vi "SDK Sample_modified.vi"() -> ()   [LabVIEW 2015]
uses:
  sub/Mode.ctl
  sub/global.vi
panel:
  out "Error?":bool
  out "size(s)":i32
  out "Data(8Bit)":u8[](array[numeric])
  out "Data(16Bit)":u16[](array[numeric])
  out "Depth":i8
  out "nDeviceNoList":u32[](array[numeric])
  out "MaxSize":cluster{"pWidth":u32, "pHeight":u32}={"pWidth"=2048, "pHeight"=2048}
  out "pDetectNumInfoLV":T1
  out "SetupCover2":string
  out "SetupCover1":string
  out "FLG_LiveStop":u16(ring) items=["Live", "Get", "Stop"]
  in  "Variable":bool caption="Calibrate"
  in  "Record Option":bool caption="Calibrate"
  in  "Update:":u16(ring) items=["OFF", "ON"]
  in  "Low  Light:":u16(ring) items=["OFF", "ON"]
  in  "Save Setup":bool caption="Calibrate"
  out "RetryCount":u8
  out "FLG_LiveStop":bool
  out "ColorType":enum16{"MONO", "COLOR"}(ring)
  out "Frame":i32(slide) scale=-2046.0..2045.0
  out "RecordStatus":u16(ring) items=["Record", "WaitingTRG", "Endless", "Recording"]
  out "Resolution":cluster{"pWidth":u32, "pHeight":u32}
  out "Picture":picture
  out "Mode":T2=enum."Error"
  out "Out_IP Address":T3 caption="Info_IP Address" {"Manual_IP"."IP4" format="%.03d"; "Manual_IP"."IP3" format="%.03d"; "Manual_IP"."IP2" format="%.03d"; "Manual_IP"."IP1" format="%.03d"; "Auto_IP"."IP3" format="%.03d"; "Auto_IP"."IP2" format="%.03d"; "Auto_IP"."IP1" format="%.03d"}
  out "nInterfaceCode":u32 format="%.0x"
  in  "stop":bool caption="停止"
  in  "Tab":enum32{"Camera", "Data Save", "File View"}(tab)
  in  "Record":bool caption="Calibrate"
  in  "RecStop":bool caption="Calibrate"
  in  "Setup":T4={"Frame Rate:"=0, "Shutter:"=0, "Resolution:"=4, "Trigger Mode:"=0, "Shading:"=0, "Partition:"=1, "Camera Option"=FALSE, "CameraInfo"={"Head:"=0, "Camera:"=0}} {"CameraInfo"."Camera:" items=["FASTCAM SA4 model 500K-M1"]; "CameraInfo"."Head:" items=["Head No.1"]; "Shading:" items=["Shading"]; "Shutter:" items=["1/50 sec", "1/60 sec", "1/100 sec", "1/200 sec", "1/300 sec", "1/400 sec", "1/500 sec", "1/600 sec", "1/700 sec", "1/800 sec", "1/900 sec", "1/1000 sec", "1/2000 sec", "1/3000 sec", "1/4000 sec", "1/5000 sec", "1/6000 sec", "1/7000 sec", "1/8000 sec", "1/9000 sec", "1/10000 sec", "1/12000 sec", "1/15000 sec", "1/17000 sec", "1/20000 sec", "1/25000 sec", "1/30000 sec", "1/34000 sec", "1/39000 sec", "1/50000 sec", "1/57000 sec", "1/62000 sec", "1/74000 sec", "1/82000 sec", "1/92000 sec", "1/104000 sec", "1/178000 sec", "1/333000 sec", "1/593000 sec", "1/1000000 sec"]; "Trigger Mode:" items=["START", "CENTER", "END", "MANUAL", "RANDOM", "RANDOM_RESET", "RANDOM_CENTER", "RANDOM_MANUAL", "TWOSTAGE_1/2", "TWOSTAGE_1/4", "TWOSTAGE_1/8"]; "Frame Rate:" items=["50 fps", "60 fps", "125 fps", "250 fps", "500 fps", "1000 fps", "2000 fps", "3000 fps", "3600 fps", "4500 fps", "5000 fps", "6000 fps", "6750 fps", "8000 fps", "10000 fps", "13500 fps", "20000 fps", "30000 fps", "40000 fps", "50000 fps", "60000 fps", "75000 fps", "86400 fps", "100000 fps", "150000 fps", "225000 fps", "360000 fps", "500000 fps"]; "Resolution:" items=["1024 X 1024", "1024 X 896", "1024 X 800", "1024 X 640", "1024 X 512", "896 X 896", "896 X 752", "896 X 640", "896 X 512", "768 X 768", "768 X 640", "768 X 512", "640 X 640", "512 X 512", "512 X 384", "512 X 352", "384 X 288", "320 X 240", "320 X 192", "320 X 160", "320 X 128", "256 X 256", "256 X 128", "256 X 64", "192 X 128", "128 X 128", "128 X 96", "128 X 64", "128 X 32", "128 X 16", "64 X 16"]; "Partition:" items=["Partition 1"=1]}
  in  "Display:":enum32{"Live", "Mem", "LiveStop"}(radio)
  in  "DataSaveInfo":T5={"DS-Format"=2, "DS-File name:"="", "DS-Save Path"=path "", "DS-Head"=0, "DS-Save"=FALSE, "Data_Slide"=0, "PLAY"=FALSE, "STOP"=FALSE, "StartFrame"=0, "EndFrame"=0, "CurrentFrame"=0, "DS-Camera:"=0} {"DS-Camera:" items=["FASTCAM SA4 model 500K-M1"]; "CurrentFrame" min=-2046 max=8871 step=1; "EndFrame" min=-2046 max=8871 step=1; "StartFrame" min=-2046 max=8871 step=1; "Data_Slide" scale=-2046.0..8871.0; "DS-Head" items=["Head No.1"]; "DS-Format" items=["BMP", "JPEG", "AVI"]}
  # "．"
  # "．"
  # "．"
  # "．"
  # "．"
  # "．"
  # "XXX"
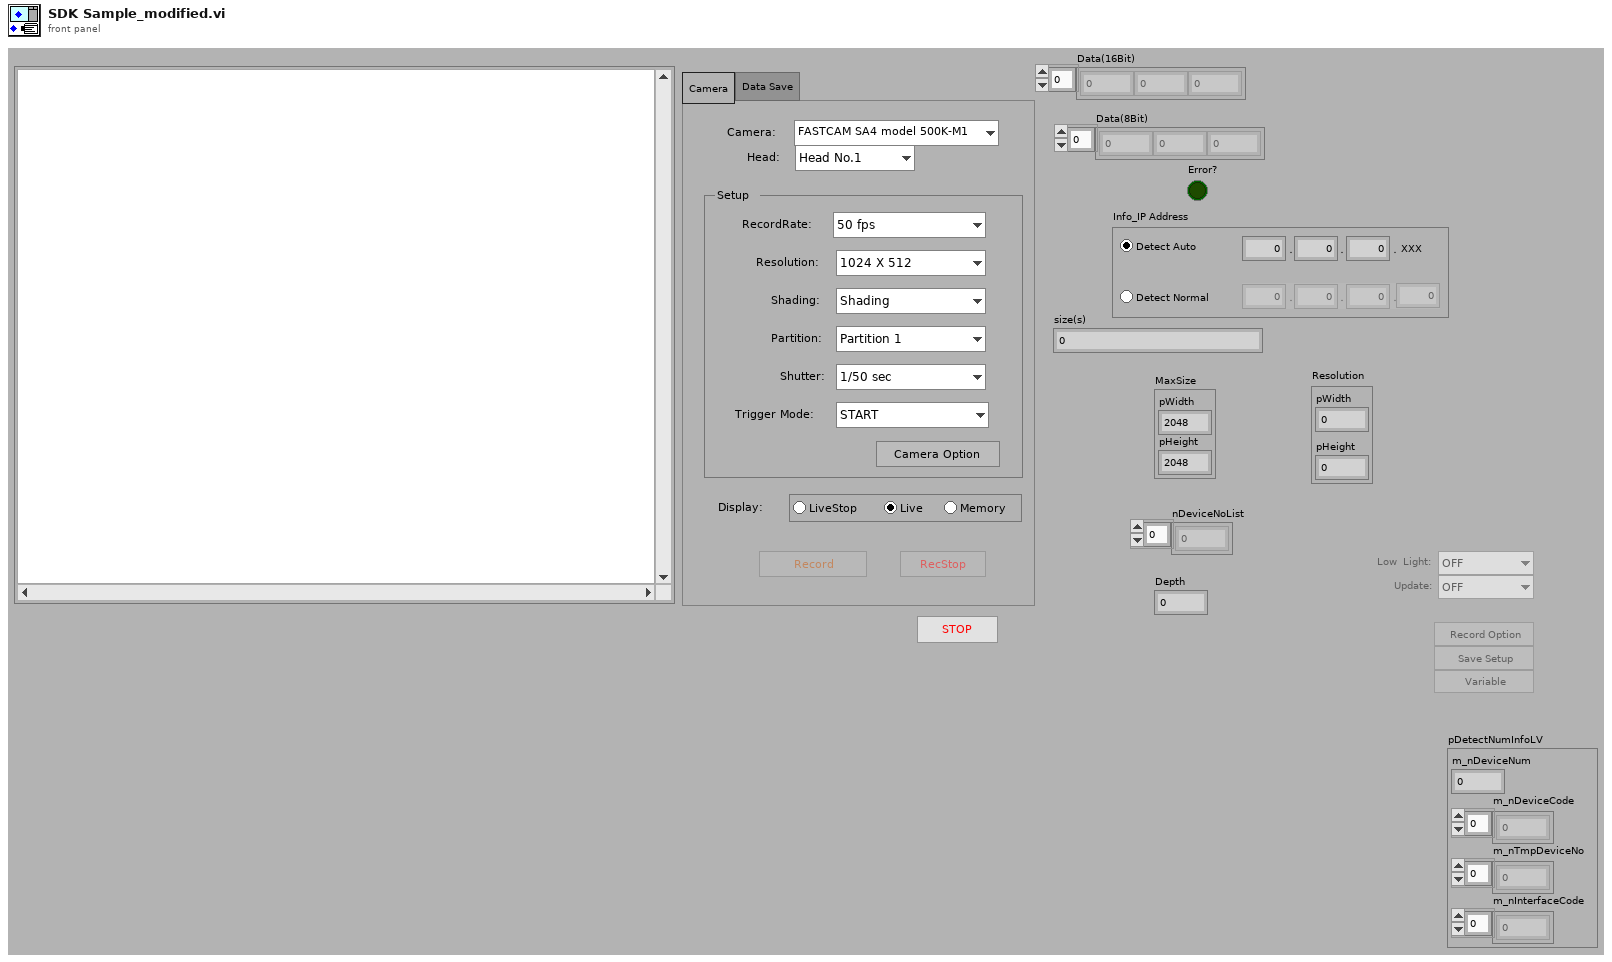
[diagram p1: front panel]
types:
  T1 = cluster{"m_nDeviceNum":u32, "m_nDeviceCode":u32[], "m_nTmpDeviceNo":u32[], "m_nInterfaceCode":u32[]}
  T2 = typedef "Mode.ctl" = enum16{"Default", "Error", "End", "Init", "DetectDevice", "Open", "Close", "GetDeviceName", "GetExistChildDeviceList", "GetColorType", "GetBitDepth.vi", "GetRecordRateList", "GetRecordRate", "SetRecordRate", "GetShutterSpeedFpsList", "GetShutterSpeedFps", "SetShutterSpeedFps", "GetResolutionList", "GetResolution", "SetResolution", "GetTriggerModeList", "GetTriggerMode", "SetTriggerMode", "GetPartitionList", "SetPartitionList", "GetCurrentPartition", "SetCurrentPartition", "GetShadingModeList", "DataSave"}
  T3 = cluster{"Detect Select BOX":enum32{"Detect Auto", "Detect Normal"}, "Auto_IP":cluster{"IP1":u8, "IP2":u8, "IP3":u8}, "Manual_IP":cluster{"IP1":u8, "IP2":u8, "IP3":u8, "IP4":u8}}
  T4 = cluster{"Frame Rate:":u16, "Shutter:":u16, "Resolution:":u16, "Trigger Mode:":u16, "Shading:":u16, "Partition:":u16, "Camera Option":bool, "CameraInfo":cluster{"Head:":u16, "Camera:":u16}}
  T5 = cluster{"DS-Format":u16, "DS-File name:":string, "DS-Save Path":path, "DS-Head":u16, "DS-Save":bool, "Data_Slide":i32, "PLAY":bool, "STOP":bool, "StartFrame":i32, "EndFrame":i32, "CurrentFrame":i32, "DS-Camera:":u16}
  T6 = enum32{"Page Enabled", "Page Disabled", "Page Disabled & Grayed"}
  T7 = cluster{"return type":u32, "pErrorCode":u32, "error ":errorcluster}
  T8 = cluster{"ReturnValue":u32, "ErrorCode":u32, "error ":errorcluster}
  T9 = cluster{"Start":i32, "End":i32, "Trigger":i32, "TwoStageLowToHigh":i32, "TwoStageHighToLow":i32, "TwoStageTiming":u32, "Event":i32[], "EventCount":u32, "RecordedFrames":u32}
  T10 = typedef "imagedata.ctl" = cluster{"image type":i32, "image depth":i32, "image":u8[], "mask":u8[], "colors":u32[], "Rectangle":cluster{"left":i16, "top":i16, "right":i16, "bottom":i16}}
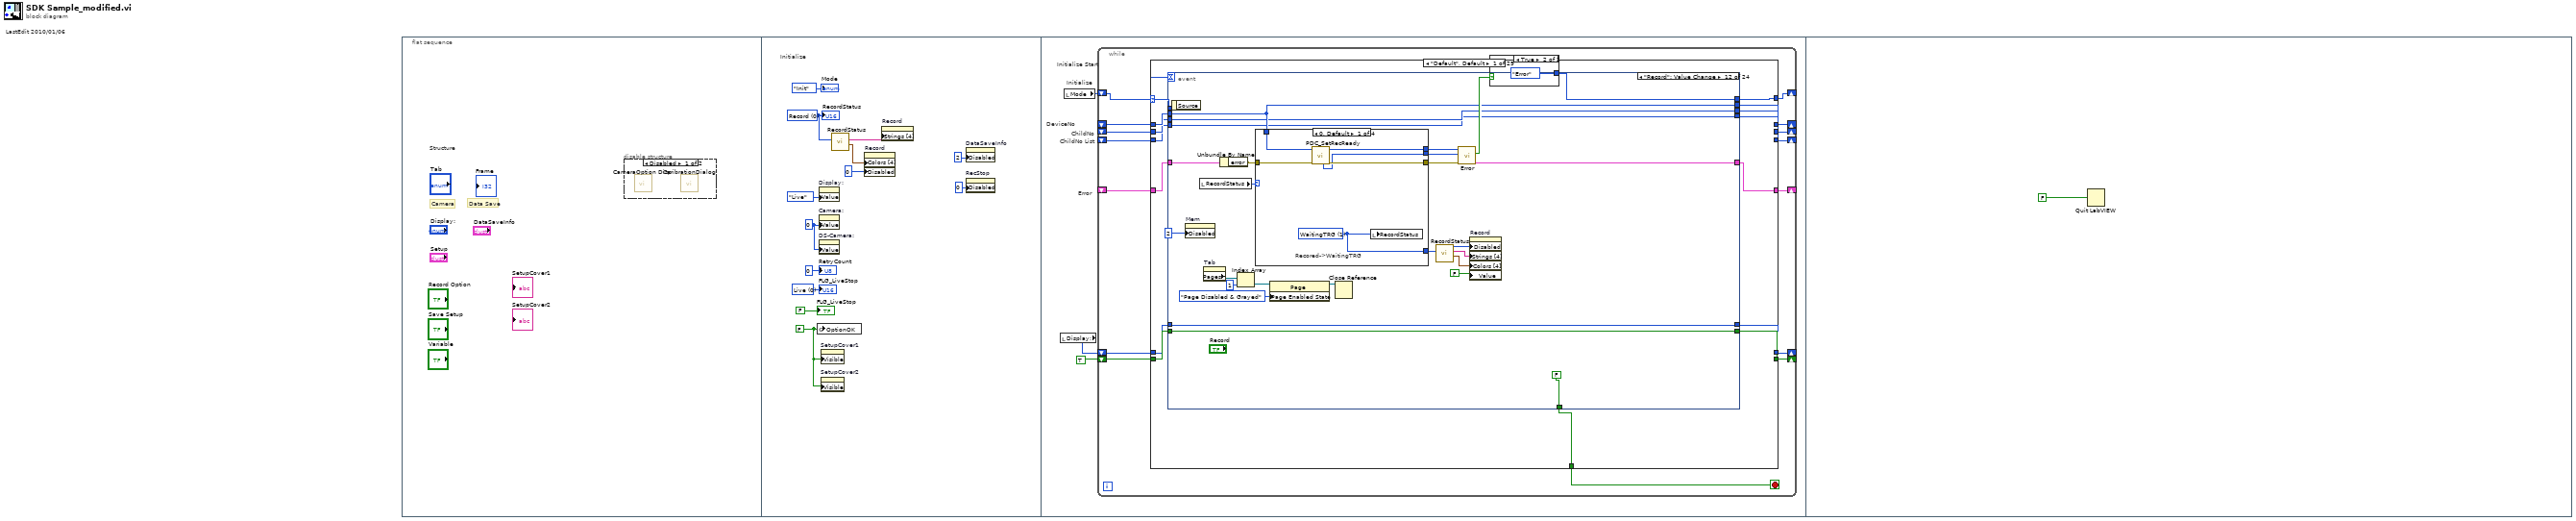
[diagram p0: block diagram]
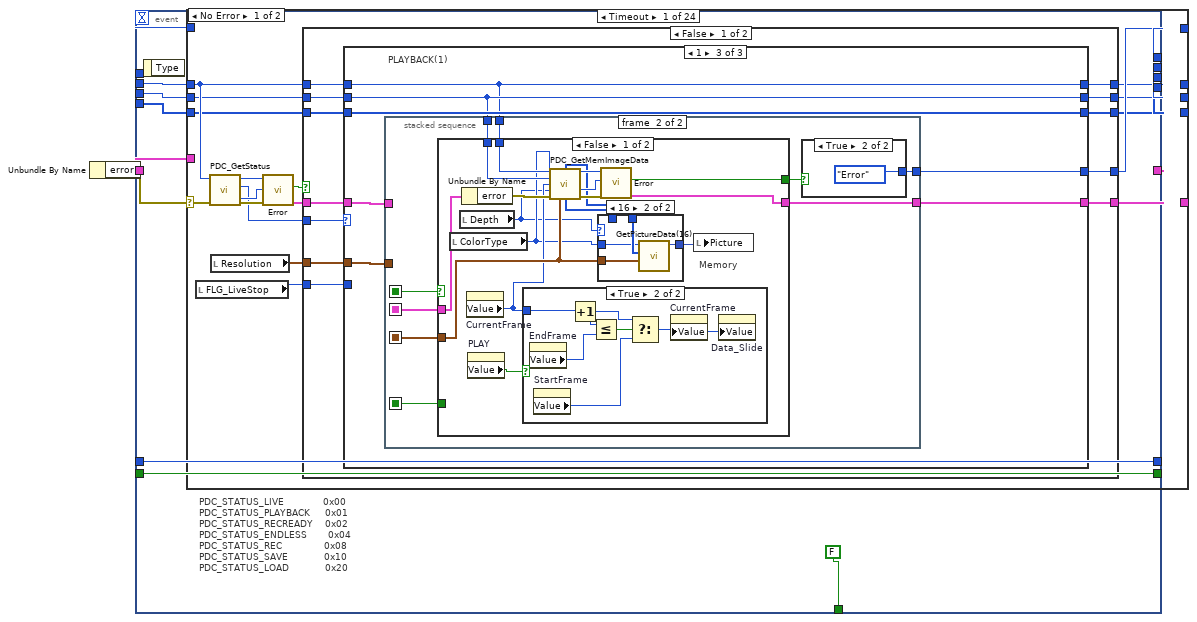
[diagram p3: hidden frame]
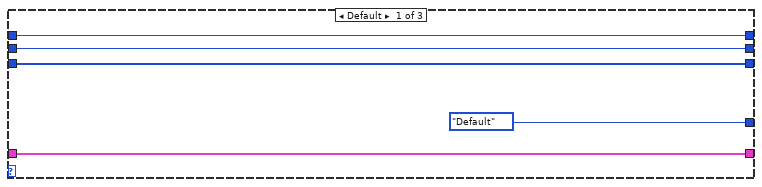
[diagram p4: hidden frame]
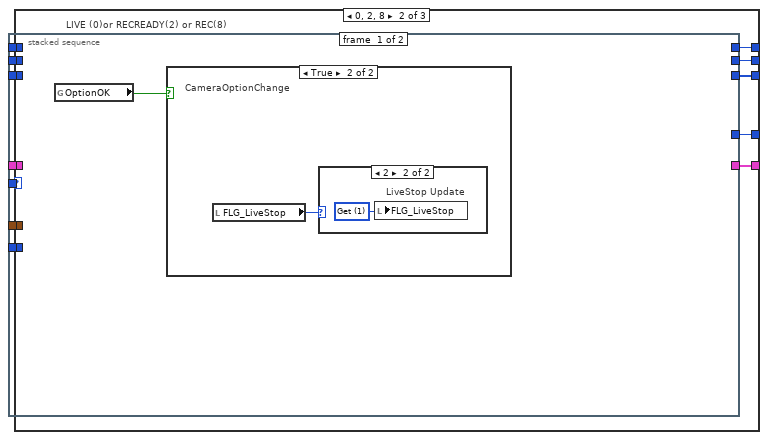
[diagram p5: hidden frame]
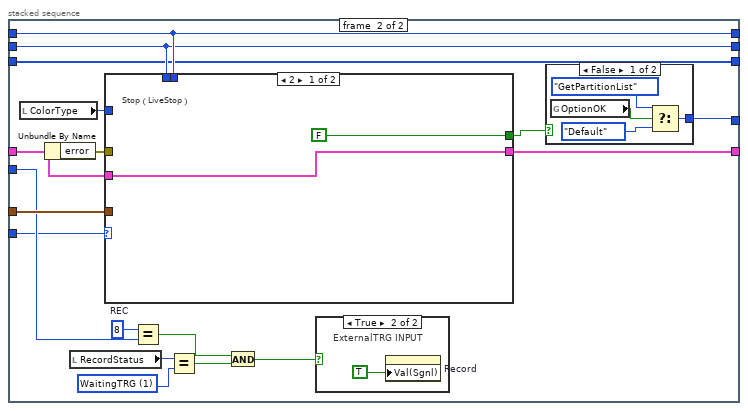
[diagram p8: hidden frame]
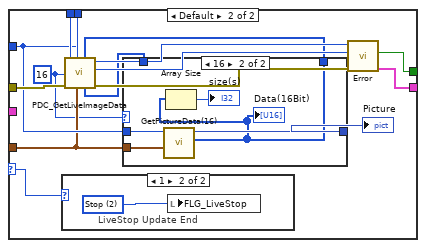
[diagram p10: hidden frame]
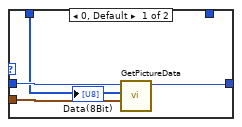
[diagram p11: hidden frame]
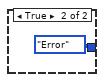
[diagram p13: hidden frame]
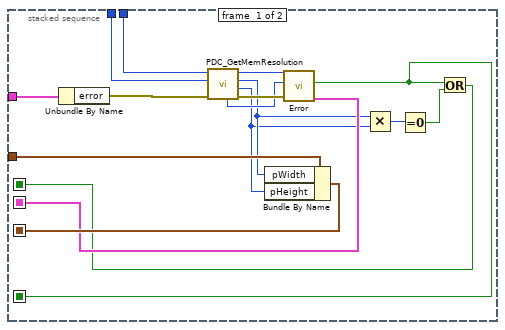
[diagram p14: hidden frame]
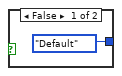
[diagram p15: hidden frame]
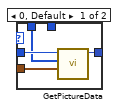
[diagram p16: hidden frame]
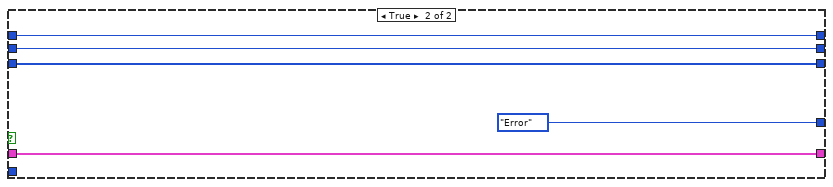
[diagram p19: hidden frame]
diagram:
  # "LastEdit 2010/01/06"
  n1 = flat-sequence {
    frame #0 {
      # "Structure"
      # "Camera"
      # "Data Save"
      n2 = disable-structure shown="Disabled" {
        frame Disabled {
          n3 = call "CameraOption Disp.vi"() -> ()  [unwired: 12 in]
          n4 = call "CaribrationDialog.vi"() -> ()  [unwired: 1 in]
        }
        frame Enabled {
        }
      }
    }
    frame #1 {
      w2 = u16 0 ("値")
      w3 = FALSE ("OptionOK")
      w4 = u16 0 items=["Live", "Get", "Stop"] ("FLG_LiveStop")
      w13 = u16 0 items=["Record", "WaitingTRG", "Endless", "Recording"] ("RecordStatus")
      # "Initialize"
      n5 = global write "global.vi" "OptionOK"(w3) -> ()
      n6 = property on="Display:" class="RadioBtnsControl (strict)"("Value"=enum32{"Live", "Mem", "LiveStop"}."Live" ("Display:")) -> ()  [unwired: 2 in, 2 out]
      n7 = property on="Camera:" class="Ring (strict)"("Value"=w2) -> ()  [unwired: 2 in, 2 out]
      n8 = property on="DS-Camera:" class="Ring (strict)"("Value"=w2) -> ()  [unwired: 2 in, 2 out]
      n9 = property on="SetupCover1" class="Str"("Visible"=w3) -> ()  [unwired: 2 in, 2 out]
      n10 = property on="SetupCover2" class="Str"("Visible"=w3) -> ()  [unwired: 2 in, 2 out]
      n11 = call "RecordStatus.vi"("RecordStatus"=w13) -> ("Color[4]"=w11:cluster{u32, u32}[], "String[4]"=w12:string[])  [unwired: 9 out]
      n12 = property on="Record" class="Bool (strict)"("Colors [4]"=w11, "Disabled"=u8 0 ("無効")) -> ()  [unwired: 2 in, 2 out]
      n13 = property on="Record" class="Bool (strict)"("Strings [4]"=w12) -> ()  [unwired: 2 in, 2 out]
      n14 = property on="DataSaveInfo" class="Clust (strict)"("Disabled"=u8 2 ("無効")) -> ()  [unwired: 2 in, 2 out]
      n15 = property on="RecStop" class="Bool (strict)"("Disabled"=u8 0 ("無効")) -> ()  [unwired: 2 in, 2 out]
      "Mode" <- Mode."Init" ("Mode")
      "RecordStatus" <- w13
      "FLG_LiveStop" <- FALSE ("FLG_LiveStop")
      "RetryCount" <- u8 0 ("RetryCount")
      "FLG_LiveStop" <- w4
    }
    frame #2 {
      # "Error"
      # "ChildNo List"
      # "Initialize"
      # "Initialize Start"
      # "ChildNo"
      # "DeviceNo"
      n16 = local read "Display:"() -> (w14:enum32{"Live", "Mem", "LiveStop"})
      n17 = local read "Mode"() -> (w16:T2)
      n18 = while {
        shift-right: [w29] -> _
        shift-left: w16 -> [w31]
        shift-right: [w27] -> _
        shift-left: _ -> [w28]
        shift-right: [w26] -> _
        shift-left: _ -> [w25]
        shift-right: [w24] -> _
        shift-left: _ -> [w23]
        shift-right: [w21] -> _
        shift-left: TRUE -> [w22]
        shift-right: [w20] -> _
        shift-left: _ -> [w19]
        shift-right: [w17] -> _
        shift-left: w14 -> [w18]
        stop <- w30 stop-if-true
        n19 = case shown="\"Default\", Default" w31 {
          selector: w31 -> [w40 _ _ _ _ _ _ _ _ _ _ _ _ _ _ _ _ _ _ _ _ _ _ _ _ _ _ _ _]
          tunnel: [w43 FALSE ("T button?") w733 FALSE ("T button?") FALSE ("T button?") FALSE ("T button?") TRUE ("T button?") FALSE ("T button?") FALSE ("T button?") FALSE ("T button?") FALSE ("T button?") FALSE ("T button?") FALSE ("T button?") FALSE ("T button?") FALSE ("T button?") FALSE ("T button?") FALSE ("T button?") FALSE ("T button?") FALSE ("T button?") FALSE ("T button?") FALSE ("T button?") FALSE ("T button?") FALSE ("T button?") FALSE ("T button?") FALSE ("T button?") FALSE ("T button?") FALSE ("T button?") FALSE ("T button?") FALSE ("T button?")] -> w30
          tunnel: w28 -> [w47 w730 w744 _ w837 w859 w894 w923 w953 w974 w991 w1012 w1040 w1065 w1088 w1118 w1142 w1171 w1207 w1240 w1260 w1283 w1301 w1335 w1357 w1379 w1391 w1418 w1467]
          tunnel: [w46 T7 {"return type"=1, "pErrorCode"=1, "error "={"status"=FALSE, "code"=0, "source"=""}} ("Error_Out") T7 {"return type"=1, "pErrorCode"=1, "error "={"status"=FALSE, "code"=0, "source"=""}} ("Error_Out") w778 w835 w858 w891 w915 w952 w972 w989 w1010 w1038 w1063 w1086 w1116 w1143 w1169 w1205 w1239 w1258 w1281 w1300 w1330 w1352 w1374 w1390 w1417 w1456] -> w27
          tunnel: [w44 Mode."Default" ("Mode") w732 w780 w838 w861 Mode."Default" ("Mode") w924 w955 w978 w995 w1016 w1044 w1069 w1092 w1122 w1144 w1175 w1211 w1237 w1264 w1286 w1299 w1329 w1351 w1373 w1394 w1403 w1454] -> w29
          tunnel: [w41 w710 w741 w774 w829 w857 w893 w921 w950 w970 w987 w1008 w1036 w1061 w1084 w1114 w1145 w1167 w1203 w1238 w1256 w1279 w1298 w1332 w1354 w1376 w1393 w1416 w1452] -> w26
          tunnel: w25 -> [w42 w710 w741 w774 w829 _ w893 w921 w950 w970 w987 w1008 w1036 w1061 w1084 w1114 w1145 w1167 w1203 w1238 w1256 w1279 w1298 w1332 w1354 w1376 w1393 w1416 w1463]
          tunnel: [w38 w711 w742 w777 w826 w856 w892 w920 w939 w966 w984 w1000 w1026 w1053 w1076 w1105 w1131 w1162 w1191 w1223 w1253 w1276 w1297 w1331 w1353 w1375 w1392 w1415 w1453] -> w24
          tunnel: w23 -> [w39 w711 w742 w777 w826 w856 w892 w920 _ w966 w984 w1000 w1026 w1053 w1076 w1105 w1131 w1162 w1191 w1223 w1253 w1276 w1297 w1331 w1353 w1375 w1392 w1415 w1468]
          tunnel: w22 -> [w37 _ _ w776 w825 w855 w890 w919 w951 w968 w986 w1002 w1028 w1052 w1075 w1104 w1130 w1161 w1190 w1222 w1250 w1273 w1292 w1326 w1349 w1371 w1388 _ w1449]
          tunnel: [w36 FALSE FALSE w776 w825 w855 w890 w919 w951 w968 w986 w1002 w1028 w1052 w1075 w1104 w1130 w1161 w1190 w1222 w1250 w1273 w1292 w1326 w1349 w1371 w1388 FALSE ("T button?") w1449] -> w21
          tunnel: [w34 w708 w739 w775 w824 w854 w889 w917 w940 w967 w985 w1001 w1027 w1051 w1074 w1103 w1129 w1160 w1189 w1221 w1249 w1271 w1291 w1325 w1348 w1370 w1387 w1406 w1447] -> w20
          tunnel: w19 -> [w35 w708 w739 w775 w824 w854 w889 w917 _ w967 w985 w1001 w1027 w1051 w1074 w1103 w1129 w1160 w1189 w1221 w1249 w1271 w1291 w1325 w1348 w1370 w1387 w1406 w1448]
          tunnel: w18 -> [w33 w707 w738 w773 w823 w853 w888 w918 w937 w965 w983 w999 w1025 w1050 w1073 w1102 w1128 w1159 w1188 w1220 w1248 w1270 w1290 w1324 w1347 w1369 w1386 w1405 w1446]
          tunnel: [w32 w707 w738 w773 w823 w853 w888 w918 w937 w965 w983 w999 w1025 w1050 w1073 w1102 w1128 w1159 w1188 w1220 w1248 w1270 w1290 w1324 w1347 w1369 w1386 w1405 w1446] -> w17
          frame "Default", Default {
            n20 = event shown="[11] \"Record\": Value Change" {
              selector: _ -> [_ _ _ _ _ _ _ _ _ _ _ _ _ _ _ _ _ _ _ _ _ _ _ _]
              dyn-events: _ -> [_ _ _ _ _ _ _ _ _ _ _ _ _ _ _ _ _ _ _ _ _ _ _ _]
              timeout: 10 -> [_ _ _ _ _ _ _ _ _ _ _ _ _ _ _ _ _ _ _ _ _ _ _ _]
              tunnel: [FALSE ("T button?") FALSE ("T button?") FALSE ("T button?") FALSE ("T button?") FALSE ("T button?") FALSE ("T button?") FALSE ("T button?") FALSE ("T button?") FALSE ("T button?") FALSE ("T button?") FALSE ("T button?") FALSE ("T button?") FALSE ("T button?") FALSE ("T button?") FALSE ("T button?") FALSE ("T button?") FALSE ("T button?") FALSE ("T button?") FALSE ("T button?") FALSE ("T button?") FALSE ("T button?") FALSE ("T button?") FALSE ("T button?") FALSE ("T button?")] -> w43
              tunnel: w47 -> [w53 w247 w258 w274 w286 w296 w306 w315 w323 w331 w361 w393 w428 w473 w555 w580 w594 w614 w638 w649 w659 w670 w686 w695]
              tunnel: [w55 w247 w258 w274 w286 w296 w306 w315 w323 w331 w361 w390 w427 w468 w555 w580 w594 w614 w638 w649 w659 w670 w686 w695] -> w46
              tunnel: [w60 w243 Mode."GetExistChildDeviceList" ("Mode") Mode."GetColorType" ("Mode") Mode."SetRecordRate" ("Mode") Mode."SetShutterSpeedFps" ("Mode") Mode."SetResolution" ("Mode") Mode."SetTriggerMode" ("Mode") Mode."SetCurrentPartition" ("Mode") w332 w358 w388 w422 w470 w559 w583 w597 w617 w634 w646 w661 Mode."GetExistChildDeviceList" ("Mode") Mode."GetColorType" ("Mode") w691] -> w44
              tunnel: w42 -> [w59 w246 _ w275 w285 w295 w305 w314 w322 w328 w359 w385 w426 w465 w558 w582 w596 w616 w635 w647 w657 _ w685 w693]
              tunnel: [w57 w246 w255 w275 w285 w295 w305 w314 w322 w328 w359 w385 w425 w466 w558 w582 w596 w616 w635 w647 w657 w668 w685 w693] -> w41
              tunnel: w40 -> [w52 _ _ _ _ _ _ _ _ w332 w358 _ _ _ w559 w583 w597 w617 w634 w646 w661 _ _ _]
              tunnel: w39 -> [w58 w242 w260 _ w282 w292 w302 w311 w320 w327 w360 w382 w424 w464 w557 w581 w595 w615 w636 w648 w658 w672 _ w692]
              tunnel: [w56 w242 w260 w270 w282 w292 w302 w311 w320 w327 w360 w382 w423 w463 w557 w581 w595 w615 w636 w648 w658 w672 w681 w692] -> w38
              tunnel: [w51 w241 TRUE ("T button?") w272 w281 w291 w301 w310 w319 w326 w356 w380 w421 w462 w560 w577 w592 w612 w633 w643 w652 TRUE ("T button?") w684 w690] -> w36
              tunnel: w37 -> [w51 w241 _ w272 w281 w291 w301 w310 w319 w326 w356 w380 w421 w462 w560 w577 w592 w612 w633 w643 w652 _ w684 w690]
              tunnel: [w49 w240 w259 w271 w280 w290 w300 w309 w318 w325 w355 w379 w419 w459 w556 w576 w591 w611 w632 w642 w651 w671 w683 w689] -> w34
              tunnel: w35 -> [w50 w240 w259 w271 w280 w290 w300 w309 w318 w325 w355 w379 w420 w460 w556 w576 w591 w611 w632 w642 w651 w671 w683 w689]
              tunnel: w33 -> [w48 w239 w261 w264 w279 w289 w299 w308 w317 w324 w354 w378 w418 w458 w552 w575 w590 w610 w631 w641 w650 w673 w675 w688]
              tunnel: [w48 w239 w261 w264 w279 w289 w299 w308 w317 w324 w354 w378 w418 w458 w553 w575 w590 w610 w631 w641 w650 w673 w675 w688] -> w32
              event Timeout {
                # "PDC_STATUS_LIVE\t\t\t\t\t\t       0x00\nPDC_STATUS_PLAYBACK\t\t\t\t\t0x01\nPDC_STATUS_RECREADY\t\t\t\t0x02\nPDC_STATUS_ENDLESS\t\t\t\t\t  0x04\nPDC_STATUS_REC\t\t\t\t\t\t        0x08\nPDC_STATUS_SAVE\t\t\t\t\t       0x10\nPDC_STATUS_LOAD\t\t\t\t\t\t      0x20"
                n21 = Unbundle By Name(w53) -> ("error"=w54:errorcluster)
                n22 = event-data() -> ()  [unwired: 2 out]
                n23 = case shown="No Error" w54 {
                  selector: w54 -> [w65 _]
                  tunnel: [w74 w235] -> w60
                  tunnel: w59 -> [w71 w237]
                  tunnel: w58 -> [w70 w236]
                  tunnel: [w69 w237] -> w57
                  tunnel: [w68 w236] -> w56
                  tunnel: [w67 w238] -> w55
                  tunnel: w53 -> [_ w238]
                  tunnel: w52 -> [_ w235]
                  tunnel: w50 -> [w64 w234]
                  tunnel: [w63 w234] -> w49
                  frame No Error {
                    n24 = local read "FLG_LiveStop"() -> (w62:u16)
                    n25 = call "PDC_GetStatus.vi"("error in (no error)"=w65, "DeviceNo"=w71) -> ("error out"=w76:errorcluster, "Status"=w73:u32, "ReturnValue"=w78:u32, "ErrorCode"=w77:u32)  [unwired: 6 out]
                    n26 = local read "Resolution"() -> (w66:cluster{"pWidth":u32, "pHeight":u32})
                    n27 = call "Error.vi"("error in (no error)"=w76, "ErrorCode"=w77, "ReturnValue"=w78) -> ("Error_Out"=w72:T8, "Error?"=w75:bool)  [unwired: 7 out]
                    n28 = case shown="False" w75 {
                      tunnel: [w83 Mode."Error" ("Mode")] -> w74
                      tunnel: w73 -> [w90 _]
                      tunnel: w72 -> [w89 w230]
                      tunnel: w71 -> [w88 w232]
                      tunnel: w70 -> [w87 w231]
                      tunnel: [w86 w232] -> w69
                      tunnel: [w85 w231] -> w68
                      tunnel: [w84 w230] -> w67
                      tunnel: w66 -> [w82 _]
                      tunnel: w64 -> [w81 w229]
                      tunnel: [w80 w229] -> w63
                      tunnel: w62 -> [w79 _]
                      frame False {
                        n29 = case shown="1" w90 {
                          selector: w90 -> [_ w102 _]
                          tunnel: w89 -> [w92 w101 w167]
                          tunnel: w88 -> [w95 w107 w162]
                          tunnel: w87 -> [w94 w106 w165]
                          tunnel: [w95 w99 w162] -> w86
                          tunnel: [w94 w98 w165] -> w85
                          tunnel: [w92 w105 w164] -> w84
                          tunnel: [Mode."Default" ("Mode") w104 w163] -> w83
                          tunnel: w82 -> [_ w103 w168]
                          tunnel: [w91 w96 w166] -> w80
                          tunnel: w81 -> [w91 w97 w166]
                          tunnel: w79 -> [_ w100 _]
                          frame Default {
                          }
                          frame 0, 2, 8 {
                            # "LIVE (0)or RECREADY(2) or REC(8)"
                            n30 = stacked-sequence {
                              tunnel: w107 -> [_ w119]
                              tunnel: w106 -> [_ w118]
                              tunnel: [_ w128] -> w105
                              tunnel: [_ w126] -> w104
                              tunnel: w103 -> [_ w125]
                              tunnel: w102 -> [_ w124]
                              tunnel: w101 -> [_ w121]
                              tunnel: w100 -> [_ w120]
                              tunnel: [_ w119] -> w99
                              tunnel: [_ w118] -> w98
                              tunnel: w97 -> [_ w117]
                              tunnel: [_ w117] -> w96
                              frame #0 {
                                n31 = global read "global.vi" "OptionOK"() -> (w108:bool)
                                n32 = case shown="True" w108 {
                                frame False {
                                }
                                frame True {
                                # "CameraOptionChange"
                                n33 = local read "FLG_LiveStop"() -> (w109:u16)
                                n34 = case shown="2" w109 {
                                frame 0, Default {
                                }
                                frame 2 {
                                w110 = u16 1 items=["Live", "Get", "Stop"] ("FLG_LiveStop")
                                # "LiveStop Update"
                                n35 = local write "FLG_LiveStop"(w110) -> ()
                                }
                                }
                                }
                                }
                              }
                              frame #1 {
                                w116 = u16 1 items=["Record", "WaitingTRG", "Endless", "Recording"] ("RecordStatus")
                                w112 = u32 8  # REC
                                n36 = local read "ColorType"() -> (w122:enum16{"MONO", "COLOR"})
                                n37 = Unbundle By Name(w121) -> ("error"=w123:errorcluster)
                                n38 = local read "RecordStatus"() -> (w115:u16)
                                n39 = case shown="2" w120 {
                                selector: w120 -> [_ w137]
                                tunnel: w119 -> [_ w146]
                                tunnel: w118 -> [_ w145]
                                tunnel: [w131 w144] -> w128
                                tunnel: [FALSE ("Error?") w143] -> w127
                                tunnel: w125 -> [_ w133]
                                tunnel: w123 -> [_ w139]
                                tunnel: w122 -> [_ w138]
                                tunnel: w121 -> [w131 _]
                                frame 2 {
                                # "Stop（LiveStop）"
                                }
                                frame Default {
                                w132 = u32 16 ("BitDepth")
                                n40 = case shown="1" w137 {
                                frame 0, Default {
                                }
                                frame 1 {
                                w156 = u16 2 items=["Live", "Get", "Stop"] ("FLG_LiveStop")
                                # "LiveStop Update End"
                                n41 = local write "FLG_LiveStop"(w156) -> ()
                                }
                                }
                                n42 = call "PDC_GetLiveImageData.vi"("Resolution"=w133, "ColorType"=w138, "error in (no error)"=w139, "BitDepth"=w132, "ChildNo"=w145, "DeviceNo"=w146) -> ("error out"=w141:errorcluster, "ErrorCode"=w136:u32, "ReturnValue"=w140:u32, "Data(8Bit)"=w135:u8[], "Data(16Bit)"=w134:u16[])  [unwired: 1 out]
                                n43 = case shown="16" w132 {
                                tunnel: w133 -> [w150 w155]
                                tunnel: [w149 w154] -> w142
                                tunnel: w134 -> [_ w151]
                                tunnel: w138 -> [w148 w153]
                                tunnel: w135 -> [w147 _]
                                frame 0, Default {
                                n44 = call "GetPictureData.vi"("Resolution"=w150, "Data(8Bit)"=w147, "ColorType"=w148) -> ("new picture"=w149:picture)  [unwired: 4 out]
                                "Data(8Bit)" <- w147
                                }
                                frame 16 {
                                n45 = call "GetPictureData(16).vi"("Resolution"=w155, "Data(16Bit)"=w151, "ColorType"=w153) -> ("new picture"=w154:picture)  [unwired: 4 out]
                                n46 = Array Size(array=w151) -> (size(s)=→"size(s)":i32)
                                "Data(16Bit)" <- w151
                                }
                                }
                                "Picture" <- w142
                                n47 = call "Error.vi"("error in (no error)"=w141, "ErrorCode"=w136, "ReturnValue"=w140) -> ("Error_Out"=w144:T8, "Error?"=w143:bool)  [unwired: 7 out]
                                }
                                }
                                n48 = Equal?(x=w112, y=w124) -> (x = y?=w114:bool)
                                n49 = Equal?(x=w115, y=w116) -> (x = y?=w113:bool)
                                n50 = And(x=w114, y=w113) -> (x .and. y?=w111:bool)
                                n51 = case shown="True" w111 {
                                frame False {
                                }
                                frame True {
                                # "ExternalTRG INPUT"
                                n52 = property on="Record" class="Bool (strict)"("Val(Sgnl)"=TRUE ("値 (信号)")) -> ()  [unwired: 2 in, 2 out]
                                }
                                }
                                n53 = case shown="False" w127 {
                                tunnel: [w157 Mode."Error" ("Mode")] -> w126
                                frame False {
                                n54 = global read "global.vi" "OptionOK"() -> (w160:bool)
                                n55 = Select(t=Mode."GetPartitionList" ("Mode"), s=w160, f=Mode."Default" ("Mode")) -> (s? t:f=w157:T2)
                                }
                                frame True {
                                }
                                }
                              }
                            }
                          }
                          frame 1 {
                            # "PLAYBACK(1)"
                            n56 = stacked-sequence {
                              seq-local: [w176 _] -> [_ w191]
                              seq-local: [w175 _] -> [_ w192]
                              seq-local: [w172 _] -> [_ w193]
                              seq-local: [w171 _] -> [_ w185]
                              tunnel: w168 -> [w179 _]
                              tunnel: w167 -> [w180 _]
                              tunnel: w162 -> [w178 w186]
                              tunnel: w165 -> [w177 w187]
                              tunnel: [_ w188] -> w164
                              tunnel: [_ w190] -> w163
                              frame #0 {
                                n57 = Unbundle By Name(w180) -> ("error"=w184:errorcluster)
                                n58 = call "PDC_GetMemResolution.vi"("error in (no error)"=w184, "ChildNo"=w177, "DeviceNo"=w178) -> ("error out"=w183:errorcluster, "Height"=w173:u32, "Width"=w174:u32, "ReturnValue"=w182:u32, "ErrorCode"=w181:u32)  [unwired: 4 in]
                                n59 = Bundle By Name(cluster=w179, "pWidth"=w174, "pHeight"=w173) -> (w176:cluster{"pWidth":u32, "pHeight":u32})
                                n60 = call "Error.vi"("error in (no error)"=w183, "ErrorCode"=w181, "ReturnValue"=w182) -> ("Error_Out"=w175:T8, "Error?"=w171:bool)  [unwired: 7 out]
                                n61 = Multiply(x=w174, y=w173) -> (x*y=w170:u32)
                                n62 = Equal To 0?(x=w170) -> (x = 0?=w169:bool)
                                n63 = Or(x=w171, y=w169) -> (x .or. y?=w172:bool)
                              }
                              frame #1 {
                                n64 = case shown="False" w193 {
                                tunnel: w192 -> [w201 w228]
                                tunnel: w191 -> [w202 _]
                                tunnel: [w204 w228] -> w188
                                tunnel: [w203 w227] -> w189
                                tunnel: w187 -> [w200 _]
                                tunnel: w186 -> [w199 _]
                                tunnel: w185 -> [_ w227]
                                frame False {
                                # "Memory"
                                n65 = local read "ColorType"() -> (w197:enum16{"MONO", "COLOR"})
                                n66 = local read "Depth"() -> (w196:i8)
                                n67 = Unbundle By Name(w201) -> ("error"=w208:errorcluster)
                                n68 = property on="CurrentFrame" class="DigNum (strict)"() -> ("Value"=w198:i32)  [unwired: 2 in, 2 out]
                                n69 = property on="PLAY" class="Bool (strict)"() -> ("Value"=w212:bool)  [unwired: 2 in, 2 out]
                                n70 = case shown="True" w212 {
                                tunnel: w198 -> [_ w226]
                                frame False {
                                }
                                frame True {
                                n71 = property on="EndFrame" class="DigNum (strict)"() -> ("Value"=w225:i32)  [unwired: 2 in, 2 out]
                                n72 = property on="StartFrame" class="DigNum (strict)"() -> ("Value"=w221:i32)  [unwired: 2 in, 2 out]
                                n73 = Increment(x=w226) -> (x+1=w222:i32)
                                n74 = Less Or Equal?(x=w222, y=w225) -> (x <= y?=w224:bool)
                                n75 = Select(t=w222, s=w224, f=w221) -> (s? t:f=w223:i32)
                                n76 = property on="CurrentFrame" class="DigNum (strict)"("Value"=w223) -> ()  [unwired: 2 in, 2 out]
                                n77 = property on="Data_Slide" class="Slide (strict)"("Value"=w223) -> ()  [unwired: 2 in, 2 out]
                                }
                                }
                                n78 = call "PDC_GetMemImageData.vi"("DeviceNo"=w199, "ColorType"=w197, "ChildNo"=w200, "FrameNo"=w198, "BitDepth"=w196, "error in (no error)"=w208, "Resolution"=w202) -> ("Data(16Bit)"=w206:u16[], "ReturnValue"=w210:u32, "Data(8Bit)"=w205:u8[], "ErrorCode"=w209:u32, "error out"=w211:errorcluster)  [unwired: 4 out]
                                n79 = case shown="16" w196 {
                                tunnel: w202 -> [w216 w220]
                                tunnel: [w215 w219] -> w207
                                tunnel: w206 -> [_ w218]
                                tunnel: w197 -> [w214 w217]
                                tunnel: w205 -> [w213 _]
                                frame 0, Default {
                                n80 = call "GetPictureData.vi"("Resolution"=w216, "Data(8Bit)"=w213, "ColorType"=w214) -> ("new picture"=w215:picture)  [unwired: 4 out]
                                }
                                frame 16 {
                                n81 = call "GetPictureData(16).vi"("Resolution"=w220, "Data(16Bit)"=w218, "ColorType"=w217) -> ("new picture"=w219:picture)  [unwired: 4 out]
                                }
                                }
                                n82 = call "Error.vi"("error in (no error)"=w211, "ErrorCode"=w209, "ReturnValue"=w210) -> ("Error_Out"=w204:T8, "Error?"=w203:bool)  [unwired: 7 out]
                                n83 = local write "Picture"(w207) -> ()
                                }
                                frame True {
                                }
                                }
                                n84 = case shown="True" w189 {
                                tunnel: [Mode."Default" ("Mode") Mode."Error" ("Mode")] -> w190
                                frame False {
                                }
                                frame True {
                                }
                                }
                              }
                            }
                          }
                        }
                      }
                      frame True {
                      }
                    }
                  }
                  frame Error {
                  }
                }
              }
              event "stop": Value Change {
                # "Program End"
                n85 = event-data() -> ()  [unwired: 2 out]
                n86 = Two Button Dialog(message="Exit the program" ("メッセージ"), 1:"CANCEL" ("Fボタン名(\"キャンセル\")"), 2:"OK" ("Tボタン名(\"OK\")")) -> (T button?=w244:bool)
                n87 = case shown="False" w244 {
                  tunnel: [Mode."Default" ("Mode") Mode."Close" ("Mode")] -> w243
                  frame False {
                  }
                  frame True {
                  }
                }
              }
              event "Setup.CameraInfo.Camera:": Value Change {
                n88 = event-data() -> ("NewVal"=w254:u16)  [unwired: 1 out]
                n89 = local read "nDeviceNoList"() -> (w257:u32[])
                n90 = property on="DS-Camera:" class="Ring (strict)"("Value"=w254) -> ()  [unwired: 2 in, 2 out]
                n91 = Index Array(array=w257, index=w254) -> (element=w255:u32)
              }
              event "Setup.CameraInfo.Head:": Value Change {
                w267 = FALSE ("PLAY")
                # "Push OK"
                n92 = event-data() -> ("NewVal"=w269:u16)  [unwired: 1 out]
                n93 = local read "FLG_LiveStop"() -> (w263:u16)
                n94 = property on="DS-Head" class="Ring (strict)"("Value"=w269) -> ()  [unwired: 2 in, 2 out]
                n95 = local read "DataSaveInfo"() -> (w268:T5)
                n96 = case shown="2" w263 {
                  frame 0, Default {
                  }
                  frame 2 {
                    w277 = u16 1 items=["Live", "Get", "Stop"] ("FLG_LiveStop")
                    # "LiveStop Update"
                    n97 = local write "FLG_LiveStop"(w277) -> ()
                  }
                }
                n98 = property on="PLAY" class="Bool (strict)"("Disabled"=u8 0 ("無効")) -> ()  [unwired: 2 in, 2 out]
                n99 = Index Array(array=w271, index=w269) -> (element=w270:u32)
                n100 = Bundle By Name(cluster=w268, "PLAY"=w267, "STOP"=w267) -> (w266:T5)
                n101 = local write "DataSaveInfo"(w266) -> ()
              }
              event "Setup.Frame Rate:": Value Change {
                # "Record Rate Change"
                n102 = event-data() -> ()  [unwired: 2 out]
                n103 = local read "FLG_LiveStop"() -> (w278:u16)
                n104 = case shown="0, Default" w278 {
                  frame 0, Default {
                  }
                  frame 2 {
                    w287 = u16 1 items=["Live", "Get", "Stop"] ("FLG_LiveStop")
                    # "LiveStop Update"
                    n105 = local write "FLG_LiveStop"(w287) -> ()
                  }
                }
              }
              event "Setup.Shutter:": Value Change {
                # "Shetter Change"
                n106 = event-data() -> ()  [unwired: 2 out]
                n107 = local read "FLG_LiveStop"() -> (w288:u16)
                n108 = case shown="2" w288 {
                  frame 0, Default {
                  }
                  frame 2 {
                    w297 = u16 1 items=["Live", "Get", "Stop"] ("FLG_LiveStop")
                    # "LiveStop Update"
                    n109 = local write "FLG_LiveStop"(w297) -> ()
                  }
                }
              }
              event "Setup.Resolution:": Value Change {
                # "Resolution Change"
                n110 = event-data() -> ()  [unwired: 2 out]
                n111 = local read "FLG_LiveStop"() -> (w298:u16)
                n112 = case shown="2" w298 {
                  frame 0, Default {
                  }
                  frame 2 {
                    w307 = u16 1 items=["Live", "Get", "Stop"] ("FLG_LiveStop")
                    # "LiveStop Update"
                    n113 = local write "FLG_LiveStop"(w307) -> ()
                  }
                }
              }
              event "Setup.Trigger Mode:": Value Change {
                # "Resolution Change"
                n114 = event-data() -> ()  [unwired: 2 out]
              }
              event "Setup.Partition:": Value Change {
                # "Resolution Change"
                n115 = event-data() -> ()  [unwired: 4 out]
              }
              event "Setup.Camera Option": Value Change {
                n116 = event-data() -> ()  [unwired: 2 out]
                n117 = flat-sequence {
                  tunnel: w328 -> [w334]
                  tunnel: w327 -> [w333]
                  tunnel: [w344] -> w329
                  tunnel: w329 -> [w349]
                  frame #0 {
                    n118 = local read "Setup"() -> (w337:T4)
                    n119 = Bundle By Name(cluster=w337, "Camera Option"=FALSE) -> (w335:T4)
                    n120 = global write "global.vi" "ChildNo"(w333) -> ()
                    n121 = global write "global.vi" "DeviceNo"(w334) -> ()
                    n122 = local write "Setup"(w335) -> ()
                  }
                  frame #1 {
                    w344 = "CameraOption Disp.vi"
                    n123 = Current VI's Path() -> (path=w348:path)
                    n124 = Strip Path(path=w348) -> (stripped path=w343:path)  [unwired: 1 out]
                    n125 = Build Path(base path=w343, name or relative path="sub") -> (appended path=w341:path)
                    n126 = property on="Camera:" class="Ring (strict)"() -> ("Strings []"=w339:string[], "Value"=w340:u16)  [unwired: 2 in, 2 out]
                    n127 = Index Array(array=w339, index=w340) -> (element=w338:string)
                    n128 = Build Path(base path=w341, name or relative path=w344) -> (appended path=w347:path)
                    n129 = Open VI Reference(vi path=w347) -> (vi reference=w346:refnum<vi>)  [unwired: 1 in, 5 out]
                    n130 = property class="VI"(reference=w346, "Front Panel.Title"=w338) -> (reference out=w345:refnum<vi>)  [unwired: 1 in, 1 out]
                    n131 = Close Reference(reference=w345) -> ()  [unwired: 1 in, 1 out]
                  }
                  frame #2 {
                    # "CALL CameraOption Disp.vi"
                    n132 = call "CallDialog.vi"("vi name"=w349) -> ()  [unwired: 3 out]
                  }
                }
              }
              event "Setup.Shading:": Mouse Down {
                n133 = event-data() -> ("CtlRef"=w353:refnum<vi>)  [unwired: 1 out]
                n134 = property class="Ring (strict)"(reference=w353) -> ("Disabled"=w352:u8)  [unwired: 1 in, 2 out]
                n135 = Equal?(x=w352, y=u8 1) -> (x = y?=w350:bool)
                n136 = case shown="True" w350 {
                  tunnel: w360 -> [_ w363]
                  tunnel: w359 -> [_ w362]
                  frame False {
                    # "Not Support"
                  }
                  frame True {
                    n137 = flat-sequence {
                      tunnel: w362 -> [w367]
                      tunnel: w363 -> [w366]
                      frame #0 {
                        n138 = local read "FLG_LiveStop"() -> (w364:u16)
                        n139 = local read "Setup"() -> (w369:T4)
                        n140 = Bundle By Name(cluster=w369, "Shading:"=u16 0 ("shading:")) -> (w368:T4)
                        n141 = case shown="2" w364 {
                          frame 0, Default {
                          }
                          frame 2 {
                            w370 = u16 1 items=["Live", "Get", "Stop"] ("FLG_LiveStop")
                            # "LiveStop Update"
                            n142 = local write "FLG_LiveStop"(w370) -> ()
                          }
                        }
                        n143 = global write "global.vi" "ChildNo"(w366) -> ()
                        n144 = global write "global.vi" "DeviceNo"(w367) -> ()
                        n145 = local write "Setup"(w368) -> ()
                      }
                      frame #1 {
                        # "CALL CaribrationDialog.vi"
                        n146 = call "CallDialog.vi"("vi name"="CaribrationDialog.vi") -> ()  [unwired: 1 in, 2 out]
                      }
                    }
                  }
                }
              }
              event "Record": Value Change {
                n147 = event-data() -> ()  [unwired: 2 out]
                n148 = property on="Mem" class="Bool (strict)"("Disabled"=u8 2 ("無効")) -> ()  [unwired: 2 in, 2 out]
                n149 = local read "RecordStatus"() -> (w396:u16)
                n150 = property on="Tab" class="TabCtl (strict)"() -> ("Pages"=w376:refnum<vi>[])  [unwired: 2 in, 2 out]
                n151 = Unbundle By Name(w393) -> ("error"=w392:errorcluster)
                n152 = Index Array(array=w376, index=1 ("指標")) -> (element=w374:refnum<vi>)
                n153 = case shown="0, Default" w396 {
                  tunnel: [w405 w411 w414 w417] -> w394
                  tunnel: w392 -> [w404 w410 w412 w416]
                  tunnel: [w403 w409 w412 w416] -> w391
                  tunnel: [w402 w408 w413 w415] -> w387
                  tunnel: [w401 w407 w413 w415] -> w386
                  tunnel: w385 -> [w400 w406 _ _]
                  frame 0, Default {
                    w405 = u16 1 items=["Record", "WaitingTRG", "Endless", "Recording"] ("RecordStatus")
                    # "Recored->WaitingTRG"
                    n154 = call "PDC_SetRecReady.vi"("error in (no error)"=w404, "DeviceNo"=w400) -> ("error out"=w403:errorcluster, "ReturnValue"=w402:u32, "ErrorCode"=w401:u32)  [unwired: 7 out]
                    n155 = local write "RecordStatus"(w405) -> ()
                  }
                  frame 1 {
                    w411 = u16 3 items=["Record", "WaitingTRG", "Endless", "Recording"] ("RecordStatus")
                    # "WaitingTRG->Recording"
                    n156 = call "PDC_TriggerIn.vi"("error in (no error)"=w410, "DeviceNo"=w406) -> ("error out"=w409:errorcluster, "ReturnValue"=w408:u32, "ErrorCode"=w407:u32)  [unwired: 7 out]
                    n157 = local write "RecordStatus"(w411) -> ()
                  }
                  frame 2 {
                    w413 = u32 1 ("return type")
                    w414 = u16 3 items=["Record", "WaitingTRG", "Endless", "Recording"] ("RecordStatus")
                    # "Endless->Recording"
                    n158 = local write "RecordStatus"(w414) -> ()
                  }
                  frame 3 {
                    w415 = u32 1 ("return type")
                    w417 = u16 3 items=["Record", "WaitingTRG", "Endless", "Recording"] ("RecordStatus")
                    # "Recording"
                    n159 = local write "RecordStatus"(w417) -> ()
                  }
                }
                n160 = property class="Page"(reference=w374, "Page Enabled State"=T6."Page Disabled & Grayed" ("ページ使用可能状態")) -> (reference out=w372:refnum<vi>)  [unwired: 1 in, 1 out]
                n161 = Close Reference(reference=w372) -> ()  [unwired: 1 in, 1 out]
                n162 = call "RecordStatus.vi"("RecordStatus"=w394) -> ("Color[4]"=w384:cluster{u32, u32}[], "String[4]"=w395:string[], "Disabled"=w383:u8)  [unwired: 8 out]
                n163 = call "Error.vi"("error in (no error)"=w391, "ErrorCode"=w386, "ReturnValue"=w387) -> ("Error_Out"=w390:T8, "Error?"=w389:bool)  [unwired: 7 out]
                n164 = property on="Record" class="Bool (strict)"("Disabled"=w383, "Strings [4]"=w395, "Colors [4]"=w384, "Value"=FALSE ("Record")) -> ()  [unwired: 2 in, 2 out]
                n165 = case shown="True" w389 {
                  tunnel: [Mode."Default" ("Mode") Mode."Error" ("Mode")] -> w388
                  frame False {
                  }
                  frame True {
                  }
                }
              }
              event "RecStop": Value Change {
                n166 = event-data() -> ()  [unwired: 2 out]
                n167 = stacked-sequence {
                  tunnel: w428 -> [_ w452]
                  tunnel: [_ w451] -> w427
                  tunnel: w426 -> [_ w450]
                  tunnel: [_ w450] -> w425
                  tunnel: w424 -> [_ w449]
                  tunnel: [_ w449] -> w423
                  tunnel: [_ w448] -> w422
                  tunnel: w420 -> [_ w441]
                  tunnel: [_ w441] -> w419
                  frame #0 {
                    w439 = u16 0 items=["Record", "WaitingTRG", "Endless", "Recording"] ("RecordStatus")
                    # "GrayScale CLEAR"
                    n168 = property on="Tab" class="TabCtl (strict)"() -> ("Pages"=w434:refnum<vi>[])  [unwired: 2 in, 2 out]
                    n169 = property on="Mem" class="Bool (strict)"("Disabled"=u8 0 ("無効")) -> ()  [unwired: 2 in, 2 out]
                    n170 = local write "RecordStatus"(w439) -> ()
                    n171 = Index Array(array=w434, index=1 ("指標")) -> (element=w432:refnum<vi>)
                    n172 = call "RecordStatus.vi"("RecordStatus"=w439) -> ("Color[4]"=w437:cluster{u32, u32}[], "String[4]"=w438:string[])  [unwired: 9 out]
                    n173 = property on="RecStop" class="Bool (strict)"("Value"=FALSE ("RecStop")) -> ()  [unwired: 2 in, 2 out]
                    n174 = property class="Page"(reference=w432, "Page Enabled State"=T6."Page Enabled" ("ページ使用可能状態")) -> (reference out=w430:refnum<vi>)  [unwired: 1 in, 1 out]
                    n175 = property on="Record" class="Bool (strict)"("Strings [4]"=w438, "Colors [4]"=w437, "Disabled"=u8 0 ("無効")) -> ()  [unwired: 2 in, 2 out]
                    n176 = Close Reference(reference=w430) -> ()  [unwired: 1 in, 1 out]
                  }
                  frame #1 {
                    w442 = u32 0  # STATUS_LIVE
                    n177 = Unbundle By Name(w452) -> ("error"=w444:errorcluster)
                    n178 = call "PDC_SetStatus.vi"("error in (no error)"=w444, "Mode"=w442, "DeviceNo"=w450) -> ("error out"=w447:errorcluster, "ReturnValue"=w446:u32, "ErrorCode"=w445:u32)  [unwired: 6 out]
                    n179 = call "Error.vi"("error in (no error)"=w447, "ErrorCode"=w445, "ReturnValue"=w446) -> ("Error_Out"=w451:T8, "Error?"=w443:bool)  [unwired: 7 out]
                    n180 = case shown="False" w443 {
                      tunnel: [Mode."Default" ("Mode") Mode."Error" ("Mode")] -> w448
                      frame False {
                      }
                      frame True {
                      }
                    }
                  }
                }
              }
              event "Display:": Value Change {
                n181 = event-data() -> ("NewVal"=w467:enum32{"Live", "Mem", "LiveStop"})  [unwired: 1 out]
                n182 = case shown="\"LiveStop\"" w467 {
                  tunnel: [u8 2 ("無効") u8 0 ("無効") u8 2 ("無効")] -> w478
                  tunnel: [w535 w542 w550] -> w472
                  tunnel: [u8 0 ("無効") u8 2 ("無効") u8 2 ("無効")] -> w456
                  tunnel: [u8 0 ("無効") u8 2 ("無効") u8 2 ("無効")] -> w461
                  tunnel: [w532 w539 w547] -> w457
                  tunnel: [FALSE w537 FALSE] -> w455
                  frame "Live", Default {
                    w532 = u16 0 items=["Live", "Get", "Stop"] ("FLG_LiveStop")
                    w535 = u32 0  # STATUS_LIVE
                    # "Live"
                  }
                  frame "Mem" {
                    w539 = u16 0 items=["Live", "Get", "Stop"] ("FLG_LiveStop")
                    w542 = u32 1  # STATUS_PLAYBACK
                    # "Memory"
                    n183 = local read "Tab"() -> (w538:enum32{"Camera", "Data Save", "File View"})
                    n184 = case shown="\"Data Save\"" w538 {
                      tunnel: [TRUE FALSE] -> w537
                      frame "Camera", Default {
                      }
                      frame "Data Save" {
                      }
                    }
                  }
                  frame "LiveStop" {
                    w547 = u16 1 items=["Live", "Get", "Stop"] ("FLG_LiveStop")
                    w550 = u32 0  # STATUS_LIVE
                    # "Memory"
                  }
                }
                n185 = local write "FLG_LiveStop"(w457) -> ()
                n186 = Unbundle By Name(w473) -> ("error"=w477:errorcluster)
                n187 = call "PDC_SetStatus.vi"("error in (no error)"=w477, "Mode"=w472, "DeviceNo"=w465) -> ("error out"=w476:errorcluster, "ReturnValue"=w475:u32, "ErrorCode"=w474:u32)  [unwired: 6 out]
                n188 = property on="DataSaveInfo" class="Clust (strict)"("Disabled"=w478) -> ()  [unwired: 2 in, 2 out]
                n189 = property on="Record" class="Bool (strict)"("Disabled"=w456) -> ()  [unwired: 2 in, 2 out]
                n190 = property on="RecStop" class="Bool (strict)"("Disabled"=w461) -> ()  [unwired: 2 in, 2 out]
                n191 = property on="SetupCover1" class="Str"("Visible"=w455) -> ()  [unwired: 2 in, 2 out]
                n192 = property on="SetupCover2" class="Str"("Visible"=w455) -> ()  [unwired: 2 in, 2 out]
                n193 = call "Error.vi"("error in (no error)"=w476, "ErrorCode"=w474, "ReturnValue"=w475) -> ("Error_Out"=w469:T8, "Error?"=w471:bool)  [unwired: 7 out]
                n194 = case shown="False" w471 {
                  tunnel: [w489 Mode."Error" ("Mode")] -> w470
                  tunnel: w469 -> [w487 w529]
                  tunnel: [w486 w529] -> w468
                  tunnel: w467 -> [w488 _]
                  tunnel: [w485 w528] -> w466
                  tunnel: w465 -> [w484 w528]
                  tunnel: w464 -> [w483 w527]
                  tunnel: [w482 w527] -> w463
                  tunnel: [w480 w526] -> w459
                  tunnel: w460 -> [w481 w526]
                  frame False {
                    n195 = case shown="\"Mem\"" w488 {
                      tunnel: [Mode."Default" ("Mode") w505] -> w489
                      tunnel: w487 -> [w493 w511]
                      tunnel: [w493 w506] -> w486
                      tunnel: [w492 w503] -> w485
                      tunnel: w484 -> [w492 w503]
                      tunnel: w483 -> [w491 w502]
                      tunnel: [w491 w502] -> w482
                      tunnel: [w490 w497] -> w480
                      tunnel: w481 -> [w490 w497]
                      frame Default {
                      }
                      frame "Mem" {
                        n196 = Unbundle By Name(w511) -> ("error"=w510:errorcluster)
                        n197 = call "PDC_GetMemFrameInfo.vi"("error in (no error)"=w510, "ChildNo"=w502, "DeviceNo"=w503) -> ("error out"=w509:errorcluster, "Frame"=w501:T9, "ReturnValue"=w508:u32, "ErrorCode"=w507:u32)  [unwired: 5 out]
                        n198 = Unbundle By Name(w501) -> ("Start"=w500:i32, "End"=w496:i32, "Trigger"=w495:i32)
                        n199 = To Double Precision Float(number=w496) -> (double precision float=w498:dbl)
                        n200 = To Double Precision Float(number=w500) -> (double precision float=w499:dbl)
                        n201 = call "Error.vi"("error in (no error)"=w509, "ErrorCode"=w507, "ReturnValue"=w508) -> ("Error_Out"=w506:T8, "Error?"=w504:bool)  [unwired: 7 out]
                        n202 = stacked-sequence {
                          tunnel: w500 -> [_ w515 _ _]
                          tunnel: w499 -> [w514 w517 w520 w523]
                          tunnel: w498 -> [w513 w516 w519 w522]
                          tunnel: w496 -> [_ _ _ w521]
                          tunnel: w495 -> [w512 _ w518 _]
                          frame #0 {
                            n203 = property on="Data_Slide" class="Slide (strict)"("Scale.Minimum"=w514, "Scale.Maximum"=w513, "Value"=w512) -> ()  [unwired: 2 in, 2 out]
                          }
                          frame #1 {
                            n204 = property on="StartFrame" class="DigNum (strict)"("Minimum"=w517, "Maximum"=w516, "Value"=w515) -> ()  [unwired: 2 in, 2 out]
                          }
                          frame #2 {
                            n205 = property on="CurrentFrame" class="DigNum (strict)"("Minimum"=w520, "Maximum"=w519, "Value"=w518) -> ()  [unwired: 2 in, 2 out]
                          }
                          frame #3 {
                            n206 = property on="EndFrame" class="DigNum (strict)"("Minimum"=w523, "Maximum"=w522, "Value"=w521) -> ()  [unwired: 2 in, 2 out]
                          }
                        }
                        n207 = case shown="False" w504 {
                          tunnel: [Mode."Default" ("Mode") Mode."Error" ("Mode")] -> w505
                          frame False {
                          }
                          frame True {
                          }
                        }
                      }
                    }
                  }
                  frame True {
                  }
                }
              }
              event "Tab": Value Change {
                n208 = event-data() -> ("NewVal"=w554:enum32{"Camera", "Data Save", "File View"})  [unwired: 1 out]
                n209 = case shown="\"Data Save\"" w554 {
                  tunnel: [w562 w572] -> w553
                  tunnel: w552 -> [w563 _]
                  frame "Camera", Default {
                    n210 = stacked-sequence {
                      tunnel: w563 -> [_ w568]
                      tunnel: [_ w568] -> w562
                      frame #0 {
                        w565 = FALSE ("PLAY")
                        # "Push OK"
                        n211 = local read "DataSaveInfo"() -> (w564:T5)
                        n212 = Bundle By Name(cluster=w564, "PLAY"=w565, "STOP"=w565) -> (w566:T5)
                        n213 = property on="PLAY" class="Bool (strict)"("Disabled"=u8 0 ("無効")) -> ()  [unwired: 2 in, 2 out]
                        n214 = local write "DataSaveInfo"(w566) -> ()
                      }
                      frame #1 {
                        n215 = case shown="\"Mem\"" w568 {
                          frame "Live", Default {
                            n216 = property on="Live" class="Bool (strict)"("Val(Sgnl)"=TRUE ("値 (信号)")) -> ()  [unwired: 2 in, 2 out]
                          }
                          frame "Mem" {
                            n217 = property on="Mem" class="Bool (strict)"("Val(Sgnl)"=TRUE ("値 (信号)")) -> ()  [unwired: 2 in, 2 out]
                          }
                          frame "LiveStop" {
                            n218 = property on="LiveStop" class="Bool (strict)"("Val(Sgnl)"=TRUE ("値 (信号)")) -> ()  [unwired: 2 in, 2 out]
                          }
                        }
                      }
                    }
                  }
                  frame "Data Save" {
                    n219 = stacked-sequence {
                      tunnel: [w573 _] -> w572
                      frame #0 {
                        n220 = property on="Display:" class="RadioBtnsControl (strict)"() -> ("Value"=w573:enum32{"Live", "Mem", "LiveStop"})  [unwired: 2 in, 2 out]
                      }
                      frame #1 {
                        n221 = property on="Mem" class="Bool (strict)"("Val(Sgnl)"=TRUE ("値 (信号)")) -> ()  [unwired: 2 in, 2 out]
                      }
                    }
                  }
                }
              }
              event "DataSaveInfo.Data_Slide": Value Change {
                n222 = event-data() -> ("NewVal"=w579:i32)  [unwired: 1 out]
                n223 = property on="CurrentFrame" class="DigNum (strict)"("Value"=w579) -> ()  [unwired: 2 in, 2 out]
              }
              event "DataSaveInfo.StartFrame": Value Change {
                n224 = property on="EndFrame" class="DigNum (strict)"() -> ("Value"=w588:i32)  [unwired: 2 in, 2 out]
                n225 = event-data() -> ("OldVal"=w584:i32, "NewVal"=w587:i32)  [unwired: 1 out]
                n226 = Less?(x=w587, y=w588) -> (x < y?=w586:bool)
                n227 = Greater Or Equal To 0?(x=w587) -> (x >= 0?=w589:bool)
                n228 = Compound Arithmetic op=AND(w589, w586) -> (w585:bool)
                n229 = case shown="True" w585 {
                  tunnel: w587 -> [_ w599]
                  tunnel: w584 -> [w598 _]
                  frame False {
                    n230 = property on="StartFrame" class="DigNum (strict)"("Value"=w598) -> ()  [unwired: 2 in, 2 out]
                  }
                  frame True {
                    n231 = property on="Data_Slide" class="Slide (strict)"() -> ("Value"=w600:i32)  [unwired: 2 in, 2 out]
                    n232 = flat-sequence {
                      tunnel: w599 -> [w603]
                      tunnel: w600 -> [w602]
                      frame #0 {
                        n233 = Greater?(x=w603, y=w602) -> (0:w604:bool)
                        n234 = Select(t=w603, s=w604, f=w602) -> (s? t:f=w601:i32)
                        n235 = property on="Data_Slide" class="Slide (strict)"("Scale.Minimum"=w603, "Value"=w601) -> ()  [unwired: 2 in, 2 out]
                        n236 = property on="CurrentFrame" class="DigNum (strict)"("Value"=w601) -> ()  [unwired: 2 in, 2 out]
                      }
                      frame #1 {
                        n237 = property on="STOP" class="Bool (strict)"("Val(Sgnl)"=TRUE ("値 (信号)")) -> ()  [unwired: 2 in, 2 out]
                      }
                    }
                  }
                }
              }
              event "DataSaveInfo.EndFrame": Value Change {
                n238 = property on="StartFrame" class="DigNum (strict)"() -> ("Value"=w608:i32)  [unwired: 2 in, 2 out]
                n239 = event-data() -> ("OldVal"=w606:i32, "NewVal"=w609:i32)  [unwired: 1 out]
                n240 = Greater?(x=w609, y=w608) -> (0:w607:bool)
                n241 = case shown="True" w607 {
                  tunnel: w609 -> [_ w619]
                  tunnel: w606 -> [w618 _]
                  frame False {
                    n242 = property on="EndFrame" class="DigNum (strict)"("Value"=w618) -> ()  [unwired: 2 in, 2 out]
                  }
                  frame True {
                    n243 = property on="Data_Slide" class="Slide (strict)"() -> ("Value"=w620:i32)  [unwired: 2 in, 2 out]
                    n244 = flat-sequence {
                      tunnel: w619 -> [w623]
                      tunnel: w620 -> [w622]
                      frame #0 {
                        n245 = Less?(x=w623, y=w622) -> (x < y?=w624:bool)
                        n246 = Select(t=w623, s=w624, f=w622) -> (s? t:f=w621:i32)
                        n247 = property on="Data_Slide" class="Slide (strict)"("Scale.Maximum"=w623, "Value"=w621) -> ()  [unwired: 2 in, 2 out]
                        n248 = property on="CurrentFrame" class="DigNum (strict)"("Value"=w621) -> ()  [unwired: 2 in, 2 out]
                      }
                      frame #1 {
                        n249 = property on="STOP" class="Bool (strict)"("Val(Sgnl)"=TRUE ("値 (信号)")) -> ()  [unwired: 2 in, 2 out]
                      }
                    }
                  }
                }
              }
              event "DataSaveInfo.CurrentFrame": Value Change {
                n250 = event-data() -> ("NewVal"=w628:i32)  [unwired: 1 out]
                n251 = property on="EndFrame" class="DigNum (strict)"() -> ("Value"=w630:i32)  [unwired: 2 in, 2 out]
                n252 = property on="StartFrame" class="DigNum (strict)"() -> ("Value"=w627:i32)  [unwired: 2 in, 2 out]
                n253 = In Range and Coerce(upper limit=w630, x=w628, lower limit=w627) -> (In Range?=w629:bool)  [unwired: 1 out]
                n254 = case shown="False" w629 {
                  tunnel: w628 -> [_ w640]
                  tunnel: [w639 w640] -> w626
                  tunnel: w627 -> [w639 _]
                  frame False {
                  }
                  frame True {
                  }
                }
                n255 = property on="CurrentFrame" class="DigNum (strict)"("Value"=w626) -> ()  [unwired: 2 in, 2 out]
                n256 = property on="Data_Slide" class="Slide (strict)"("Value"=w626) -> ()  [unwired: 2 in, 2 out]
              }
              event "DataSaveInfo.PLAY": Value Change {
                # "No Push"
                n257 = event-data() -> ()  [unwired: 7 out]
                n258 = property on="PLAY" class="Bool (strict)"("Disabled"=u8 1 ("無効")) -> ()  [unwired: 2 in, 2 out]
              }
              event "DataSaveInfo.STOP": Value Change {
                w655 = FALSE ("PLAY")
                # "Push OK"
                n259 = event-data() -> ()  [unwired: 2 out]
                n260 = local read "DataSaveInfo"() -> (w656:T5)
                n261 = Bundle By Name(cluster=w656, "PLAY"=w655, "STOP"=w655) -> (w654:T5)
                n262 = property on="PLAY" class="Bool (strict)"("Disabled"=u8 0 ("無効")) -> ()  [unwired: 2 in, 2 out]
                n263 = local write "DataSaveInfo"(w654) -> ()
              }
              event "DataSaveInfo.DS-Camera:": Value Change {
                w665 = FALSE ("PLAY")
                n264 = event-data() -> ("NewVal"=w663:u16)  [unwired: 1 out]
                n265 = local read "DataSaveInfo"() -> (w666:T5)
                n266 = Bundle By Name(cluster=w666, "PLAY"=w665, "STOP"=w665) -> (w664:T5)
                n267 = local write "DataSaveInfo"(w664) -> ()
                n268 = local read "nDeviceNoList"() -> (w669:u32[])
                n269 = Index Array(array=w669, index=w663) -> (element=w668:u32)
                n270 = property on="Camera:" class="Ring (strict)"("Value"=w663) -> ()  [unwired: 2 in, 2 out]
              }
              event "DataSaveInfo.DS-Head": Value Change {
                w678 = FALSE ("PLAY")
                # "Push OK"
                n271 = event-data() -> ("NewVal"=w680:u16)  [unwired: 1 out]
                n272 = property on="Head:" class="Ring (strict)"("Value"=w680) -> ()  [unwired: 2 in, 2 out]
                n273 = local read "DataSaveInfo"() -> (w679:T5)
                n274 = Index Array(array=w683, index=w680) -> (element=w681:u32)
                n275 = Bundle By Name(cluster=w679, "PLAY"=w678, "STOP"=w678) -> (w677:T5)
                n276 = property on="PLAY" class="Bool (strict)"("Disabled"=u8 0 ("無効")) -> ()  [unwired: 2 in, 2 out]
                n277 = local write "DataSaveInfo"(w677) -> ()
              }
              event "DataSaveInfo.DS-Save": Value Change {
                n278 = flat-sequence {
                  tunnel: [w697] -> w691
                  frame #0 {
                    n279 = property on="DS-Save" class="Bool (strict)"("Value"=FALSE ("値")) -> ()  [unwired: 2 in, 2 out]
                  }
                  frame #1 {
                    n280 = local read "DataSaveInfo"() -> (w703:T5)
                    n281 = Unbundle By Name(w703) -> ("DS-Save Path"=w702:path, "DS-File name:"=w701:string)
                    n282 = Build Path(base path=w702, name or relative path=w701) -> (appended path=w700:path)
                    n283 = Not Equal?(x=w700, y=path "") -> (x != y?=w698:bool)
                    n284 = case shown="False" w698 {
                      tunnel: [Mode."Default" ("Mode") Mode."DataSave" ("Mode")] -> w697
                      frame False {
                        n285 = One Button Dialog(message="Filename Error" ("メッセージ")) -> ()  [unwired: 2 out]
                      }
                      frame True {
                      }
                    }
                  }
                }
                n286 = event-data() -> ()  [unwired: 2 out]
              }
            }
          }
          frame "Error" {
            w712 = "\r\n"
            n287 = Unbundle By Name(w730) -> ("error"=w728:errorcluster, "error.source"=w725:string, "error.code"=w724:i32, "ReturnValue"=w721:u32, "ErrorCode"=w720:u32)
            n288 = Number To Decimal String(number=w724) -> (decimal integer string=w722:string)  [unwired: 1 out]
            n289 = Number To Decimal String(number=w721) -> (decimal integer string=w718:string)  [unwired: 1 out]
            n290 = Number To Decimal String(number=w720) -> (decimal integer string=w716:string)  [unwired: 1 out]
            n291 = call <vilib>:"Clear Errors.vi"("error in (no error)"=w728) -> ("error out"=w727:errorcluster)  [unwired: 1 in, 5 out]
            n292 = Concatenate Strings("<<Error !!>>", w712, w712, w712, "Source=", w725, w712, "LabError=", w722, w712, "ReturnType=", w718, w712, "ErrorCode=", w716) -> (w715:string)
            n293 = call "メッセージ表示"("error in (no error)"=w727, "Message"=w715) -> ()  [unwired: 1 in, 9 out]
          }
          frame "End" {
            n294 = local read "RetryCount"() -> (w737:u8)
            n295 = Increment(x=w737) -> (x+1=w736:u8)
            n296 = Greater Or Equal?(x=w736, y=u8 3) -> (x >= y?=w734:bool)
            n297 = local write "RetryCount"(w736) -> ()
            n298 = case shown="True" w734 {
              tunnel: w744 -> [_ w765]
              tunnel: [FALSE ("T button?") TRUE ("T button?")] -> w733
              tunnel: [Mode."Init" ("Mode") Mode."Default" ("Mode")] -> w732
              frame False {
                # "Retry"
              }
              frame True {
                w749 = "\r\n"
                n299 = Unbundle By Name(w765) -> ("error"=w764:errorcluster, "error.source"=w761:string, "error.code"=w760:i32, "ReturnValue"=w757:u32, "ErrorCode"=w756:u32)
                n300 = Number To Decimal String(number=w760) -> (decimal integer string=w758:string)  [unwired: 1 out]
                n301 = Number To Decimal String(number=w757) -> (decimal integer string=w754:string)  [unwired: 1 out]
                n302 = Number To Decimal String(number=w756) -> (decimal integer string=w752:string)  [unwired: 1 out]
                n303 = call <vilib>:"Clear Errors.vi"("error in (no error)"=w764) -> ("error out"=w763:errorcluster)  [unwired: 1 in, 5 out]
                n304 = Concatenate Strings("<<Error !!>>", w749, w749, w749, "Source=", w761, w749, "LabError=", w758, w749, "ReturnType=", w754, w749, "ErrorCode=", w752) -> (w751:string)
                n305 = call "メッセージ表示2"("error in (no error)"=w763, "Message"=w751) -> ()  [unwired: 1 in, 9 out]
              }
            }
          }
          frame "Init" {
            w768 = u32 1 ("return type")
            # "PDC_INTTYPE_G_ETHER\t\t\t0x00000002\nPDC_INTTYPE_IEEE1394\t\t\t0x00000003\nPDC_INTTYPE_PCI\t\t\t\t\t\t     0x00000100"
            n306 = call "InterfaceSelect.vi"("error in (no error)"=errorcluster {"status"=FALSE, "code"=0, "source"=""}) -> ("error out"=w769:errorcluster, "Out_IP Address"=→"Out_IP Address":T3, "nInterfaceCode"=→"nInterfaceCode":u32)  [unwired: 1 in, 7 out]
            n307 = call "Error.vi"("error in (no error)"=w769, "ErrorCode"=w768, "ReturnValue"=w768) -> ("Error_Out"=w767:T8, "Error?"=w766:bool)  [unwired: 7 out]
            "Error?" <- w766
            n308 = case shown="False" w766 {
              tunnel: [w788 TRUE ("Error?")] -> w779
              tunnel: [w786 w799] -> w778
              tunnel: w774 -> [w784 _]
              tunnel: w767 -> [w783 w799]
              frame False {
                n309 = Unbundle By Name(w783) -> ("error"=w787:errorcluster)
                n310 = call "PDC_Init.vi"("error in (no error)"=w787) -> ("error out"=w789:errorcluster, "ErrorCode"=w785:u32, "ReturnValue"=w782:u32)  [unwired: 8 out]
                n311 = case shown="7" w785 {
                  tunnel: w789 -> [w790 w798]
                  tunnel: w782 -> [_ w797]
                  tunnel: [FALSE ("Error?") w796] -> w788
                  tunnel: [T7 {"return type"=1, "pErrorCode"=1, "error "={"status"=FALSE, "code"=0, "source"=""}} ("Error_Out") w795] -> w786
                  tunnel: w785 -> [_ w794]
                  tunnel: w784 -> [w791 _]
                  frame 7 {
                    # "既に初期化済み"
                    n312 = call "PDC_CloseDevice.vi"("error in (no error)"=w790, "DeviceNo"=w791) -> ()  [unwired: 3 in, 7 out]
                  }
                  frame Default {
                    n313 = call "Error.vi"("error in (no error)"=w798, "ErrorCode"=w794, "ReturnValue"=w797) -> ("Error_Out"=w795:T8, "Error?"=w796:bool)  [unwired: 7 out]
                  }
                }
              }
              frame True {
              }
            }
            n314 = case shown="False" w779 {
              tunnel: [Mode."DetectDevice" ("Mode") Mode."Error" ("Mode")] -> w780
              frame False {
              }
              frame True {
              }
            }
          }
          frame "DetectDevice" {
            w816 = TRUE  # NoSearch
            # "PDC_DetectDeviceLV"
            # "IP Address\nReplace"
            n315 = local read "Out_IP Address"() -> (w828:T3)
            n316 = global read "global.vi" "PDC_MAX_DEVICE"() -> (w806:i32)
            n317 = Unbundle By Name(w828) -> ("Detect Select BOX"=w827:enum32{"Detect Auto", "Detect Normal"})
            n318 = local read "nInterfaceCode"() -> (w809:u32)
            n319 = case shown="\"Detect Auto\", Default" w827 {
              tunnel: [u32 1 u32 0] -> w803
              frame "Detect Auto", Default {
              }
              frame "Detect Normal" {
              }
            }
            n320 = call "GetIPString.vi"("Out_IP Address"=w828) -> ("Net address"=w831:u32)  [unwired: 10 out]
            n321 = Initialize Array "Initialize Array"(u32 0 ("要素"), w806) -> (w833:u32[])
            n322 = Equal?(x=2, y=w809) -> (x = y?=w807:bool)
            n323 = Replace Array Subset "Replace Array Subset"(array=w833, new element=w831, index=0 ("指標")) -> (w830:u32[])
            n324 = Unbundle By Name(w837) -> ("error"=w836:errorcluster)
            n325 = Select(t=1, s=w807, f=w806) -> (s? t:f=w804:i32)
            n326 = call "PDC_DetectDevice.vi"("InterfaceCode"=w809, "DetectNum"=w804, "DetectParam"=w803, "error in (no error)"=w836, "DetectNo"=w830) -> ("DeviceNum"=w815:u32, "ReturnValue"=w821:u32, "DeviceCode"=w813:u32[], "TmpDeviceNo"=w812:u32[], "InterfaceCode(out)"=w811:u32[], "ErrorCode"=w820:u32, "error out"=w822:errorcluster)  [unwired: 1 in, 3 out]
            n327 = local read "pDetectNumInfoLV"() -> (w814:T1)
            n328 = Bundle By Name(cluster=w814, "m_nDeviceNum"=w815, "m_nDeviceCode"=w813, "m_nTmpDeviceNo"=w812, "m_nInterfaceCode"=w811) -> (→"pDetectNumInfoLV":T1)
            n329 = call "Error.vi"("error in (no error)"=w822, "ErrorCode"=w820, "ReturnValue"=w821) -> ("Error_Out"=w835:T8, "Error?"=w818:bool)  [unwired: 7 out]
            n330 = Equal To 0?(x=w815) -> (x = 0?=w819:bool)
            n331 = Select(t=w816, s=w819, f=w818) -> (s? t:f=w817:bool)
            n332 = case shown="False" w817 {
              tunnel: [Mode."Open" ("Mode") Mode."End" ("Mode")] -> w838
              frame False {
              }
              frame True {
                # "Retry 3times"
              }
            }
          }
          frame "Open" {
            # "<-OpenOK\n   DeviceList"
            # "DeviceSelect"
            # "ALL DeviceError->"
            # "PDC_DetectDeviceLV"
            n333 = local read "pDetectNumInfoLV"() -> (w851:T1)
            n334 = Unbundle By Name(w851) -> ("m_nDeviceNum"=w850:u32, "m_nDeviceCode"=w849:u32[], "m_nTmpDeviceNo"=w848:u32[], "m_nInterfaceCode"=w847:u32[])
            n335 = for {
              N: w850 -> [_]
              tunnel: [w866] -> w845 mode=indexing
              shift-right: [w878] -> w858
              shift-left: w859 -> [w879]
              tunnel: w849 -> [w873]
              tunnel: w848 -> [w872]
              tunnel: w847 -> [w871]
              shift-right: [w863] -> w852
              shift-left: u32[] [] ("nDeviceNoList") -> [w865]
              i -> [w870]
              n336 = Unbundle By Name(w879) -> ("error"=w875:errorcluster)
              n337 = Index Array(array=w873, index=w870) -> (element=w869:u32)
              n338 = Index Array(array=w872, index=w870) -> (element=w868:u32)
              n339 = Index Array(array=w871, index=w870) -> (element=w867:u32)
              n340 = call "PDC_OpenDevice.vi"("error in (no error)"=w875, "InterfaceCode"=w867, "TmpDeviceNo"=w868, "DeviceCode"=w869) -> ("error out"=w877:errorcluster, "DeviceNo"=w864:u32, "ErrorCode"=w874:u32, "ReturnValue"=w876:u32)  [unwired: 4 out]
              n341 = call "Error.vi"("error in (no error)"=w877, "ErrorCode"=w874, "ReturnValue"=w876) -> ("Error_Out"=w878:T8, "Error?"=w866:bool)  [unwired: 7 out]
              n342 = case shown="False" w866 {
                tunnel: w865 -> [w882 w883]
                tunnel: w864 -> [w881 _]
                tunnel: [w880 w883] -> w863
                frame False {
                  n343 = Build Array (concatenate)(w882, w881) -> (w880:u32[])
                }
                frame True {
                  # "NoDevice"
                }
              }
            }
            "nDeviceNoList" <- w852
            n344 = property on="Camera:" class="Ring (strict)"() -> ("Value"=w846:u16)  [unwired: 2 in, 2 out]
            n345 = And Array Elements(Boolean array=w845) -> (logical AND=w860:bool)
            n346 = Index Array(array=w852, index=w846) -> (element=w857:u32)
            n347 = case shown="True" w860 {
              tunnel: [Mode."GetDeviceName" ("Mode") Mode."End" ("Mode")] -> w861
              frame False {
                n348 = local write "RetryCount"(u8 0 ("RetryCount")) -> ()
              }
              frame True {
              }
            }
          }
          frame "Close" {
            n349 = local read "nDeviceNoList"() -> (w887:u32[])
            n350 = for {
              tunnel: w887 -> [w897] mode=indexing
              shift-right: [w898] -> w891
              shift-left: w894 -> [w907]
              n351 = Unbundle By Name(w907) -> ("error"=w906:errorcluster)
              n352 = call "PDC_CloseDevice.vi"("error in (no error)"=w906, "DeviceNo"=w897) -> ("error out"=w901:errorcluster, "ErrorCode"=w905:u32, "ReturnValue"=w908:u32)  [unwired: 3 in, 4 out]
              n353 = call "Error.vi"("error in (no error)"=w901, "ErrorCode"=w905, "ReturnValue"=w908) -> ("Error_Out"=w900:T8)  [unwired: 8 out]
              n354 = local read "nInterfaceCode"() -> (w903:u32)
              n355 = local read "Out_IP Address"() -> (w902:T3)
              n356 = call "Interface_RW.vi"("Mode"=enum16{"Write", "Read"}."Write", "error in (no error)"=w901, "In_IP Address"=w902, "In_InterfaceCode"=w903) -> ("error out"=w899:errorcluster)  [unwired: 7 out]
              n357 = Bundle By Name(cluster=w900, "error"=w899) -> (w898:T8)
            }
          }
          frame "GetDeviceName" {
            n358 = Unbundle By Name(w923) -> ("error"=w922:errorcluster)
            n359 = local read "nDeviceNoList"() -> (w909:u32[])
            n360 = for {
              tunnel: w909 -> [w926] mode=indexing
              tunnel: [w933] -> w916 mode=indexing
              shift-right: [w932] -> _
              shift-left: w922 -> [w934]
              tunnel: [w931] -> w915
              tunnel: [w928] -> w914 mode=indexing
              w927 = u32 0  # Device (Main set)
              n361 = call "PDC_GetDeviceName.vi"("error in (no error)"=w934, "ChildNo"=w927, "DeviceNo"=w926) -> ("error out"=w932:errorcluster, "StrName"=w933:string, "ReturnValue"=w930:u32, "ErrorCode"=w929:u32)  [unwired: 1 in, 4 out]
              n362 = call "Error.vi"("error in (no error)"=w932, "ErrorCode"=w929, "ReturnValue"=w930) -> ("Error_Out"=w931:T8, "Error?"=w928:bool)  [unwired: 7 out]
            }
            n363 = Search 1D Array(1D array=w914, element=TRUE ("要素")) -> (index of element=w912:i32)  [unwired: 1 out]
            n364 = property on="Camera:" class="Ring (strict)"("Strings []"=w916) -> ()  [unwired: 2 in, 2 out]
            n365 = property on="DS-Camera:" class="Ring (strict)"("Strings []"=w916) -> ()  [unwired: 2 in, 2 out]
            n366 = Not Equal?(x=w912, y=-1) -> (x != y?=w910:bool)
            n367 = case shown="False" w910 {
              tunnel: [Mode."GetExistChildDeviceList" ("Mode") Mode."Error" ("Mode")] -> w924
              frame False {
              }
              frame True {
              }
            }
          }
          frame "GetExistChildDeviceList" {
            w941 = u32 0 ("値")
            n368 = Unbundle By Name(w953) -> ("error"=w947:errorcluster)
            n369 = call "PDC_GetExistChildDeviceList.vi"("error in (no error)"=w947, "DeviceNo"=w950) -> ("error out"=w948:errorcluster, "List"=w940:u32[], "Size"=w946:u32, "ReturnValue"=w949:u32, "ErrorCode"=w942:u32)  [unwired: 5 out]
            n370 = for {
              N: w946 -> [_]
              tunnel: "Head No." -> [w962]
              tunnel: "%d" -> [w961]
              tunnel: [w960] -> w943 mode=indexing
              tunnel: w940 -> [w959]
              i -> [w958]
              n371 = Index Array(array=w959, index=w958) -> (element=w957:u32)
              n372 = Format Value(string ("")=w962, format string=w961, value (0)=w957) -> (output string=w960:string)
            }
            n373 = Index Array(array=w940, index=0 ("指標")) -> (element=w939:u32)
            n374 = property on="Head:" class="Ring (strict)"("Strings []"=w943, "Value"=w941) -> ()  [unwired: 2 in, 2 out]
            n375 = property on="DS-Head" class="Ring (strict)"("Strings []"=w943, "Value"=w941) -> ()  [unwired: 2 in, 2 out]
            n376 = call "Error.vi"("error in (no error)"=w948, "ErrorCode"=w942, "ReturnValue"=w949) -> ("Error_Out"=w952:T8, "Error?"=w954:bool)  [unwired: 7 out]
            n377 = case shown="False" w954 {
              tunnel: [Mode."GetColorType" ("Mode") Mode."Error" ("Mode")] -> w955
              frame False {
              }
              frame True {
              }
            }
          }
          frame "GetColorType" {
            # "PDC_COLORTYPE_MONO\t\t\t\t\t0\nPDC_COLORTYPE_COLOR\t\t\t\t1"
            n378 = Unbundle By Name(w974) -> ("error"=w973:errorcluster)
            n379 = call "PDC_GetColorType.vi"("error in (no error)"=w973, "ChildNo"=w966, "DeviceNo"=w970) -> ("error out"=w977:errorcluster, "Mode"=→"ColorType":i8, "ReturnValue"=w976:u32, "ErrorCode"=w971:u32)  [unwired: 5 out]
            n380 = call "Error.vi"("error in (no error)"=w977, "ErrorCode"=w971, "ReturnValue"=w976) -> ("Error_Out"=w972:T8, "Error?"=w975:bool)  [unwired: 7 out]
            n381 = case shown="False" w975 {
              tunnel: [Mode."GetBitDepth.vi" ("Mode") Mode."Error" ("Mode")] -> w978
              frame False {
              }
              frame True {
              }
            }
          }
          frame "GetBitDepth.vi" {
            n382 = Unbundle By Name(w991) -> ("error"=w990:errorcluster)
            n383 = call "PDC_GetBitDepth.vi"("error in (no error)"=w990, "ChildNo"=w984, "DeviceNo"=w987) -> ("error out"=w994:errorcluster, "Depth"=→"Depth":i8, "ReturnValue"=w993:u32, "ErrorCode"=w988:u32)  [unwired: 5 out]
            n384 = call "Error.vi"("error in (no error)"=w994, "ErrorCode"=w988, "ReturnValue"=w993) -> ("Error_Out"=w989:T8, "Error?"=w992:bool)  [unwired: 7 out]
            n385 = case shown="False" w992 {
              tunnel: [Mode."GetRecordRateList" ("Mode") Mode."Error" ("Mode")] -> w995
              frame False {
              }
              frame True {
              }
            }
          }
          frame "GetRecordRateList" {
            n386 = Unbundle By Name(w1012) -> ("error"=w1011:errorcluster)
            n387 = call "PDC_GetRecordRateList.vi"("error in (no error)"=w1011, "ChildNo"=w1000, "DeviceNo"=w1008) -> ("error out"=w1015:errorcluster, "List"=w1007:u32[], "Size"=w1003:u32, "ReturnValue"=w1014:u32, "ErrorCode"=w1009:u32)  [unwired: 4 out]
            n388 = Number To Decimal String(number=w1007) -> (decimal integer string=w1006:string[])  [unwired: 1 out]
            n389 = for {
              N: w1003 -> [_]
              tunnel: w1006 -> [w1020]
              tunnel: [w1022] -> w1005 mode=indexing
              tunnel: " fps" -> [w1021]
              i -> [w1019]
              n390 = Index Array(array=w1020, index=w1019) -> (element=w1018:string)
              n391 = Concatenate Strings(w1018, w1021) -> (w1022:string)
            }
            n392 = call "Error.vi"("error in (no error)"=w1015, "ErrorCode"=w1009, "ReturnValue"=w1014) -> ("Error_Out"=w1010:T8, "Error?"=w1013:bool)  [unwired: 7 out]
            n393 = property on="Frame Rate:" class="Ring (strict)"("Strings []"=w1005) -> ()  [unwired: 2 in, 2 out]
            n394 = case shown="False" w1013 {
              tunnel: [Mode."GetRecordRate" ("Mode") Mode."Error" ("Mode")] -> w1016
              frame False {
              }
              frame True {
              }
            }
          }
          frame "GetRecordRate" {
            n395 = Unbundle By Name(w1040) -> ("error"=w1039:errorcluster)
            n396 = call "PDC_GetRecordRate.vi"("error in (no error)"=w1039, "ChildNo"=w1026, "DeviceNo"=w1036) -> ("error out"=w1043:errorcluster, "Rate"=w1034:u32, "ReturnValue"=w1042:u32, "ErrorCode"=w1037:u32)  [unwired: 5 out]
            n397 = Number To Decimal String(number=w1034) -> (decimal integer string=w1033:string)  [unwired: 1 out]
            n398 = property on="Frame Rate:" class="Ring (strict)"() -> ("Strings []"=w1032:string[])  [unwired: 2 in, 2 out]
            n399 = Concatenate Strings(w1033, " fps") -> (w1031:string)
            n400 = call "Error.vi"("error in (no error)"=w1043, "ErrorCode"=w1037, "ReturnValue"=w1042) -> ("Error_Out"=w1038:T8, "Error?"=w1041:bool)  [unwired: 7 out]
            n401 = Search 1D Array(1D array=w1032, element=w1031) -> (index of element=w1030:i32)  [unwired: 1 out]
            n402 = case shown="-1" w1030 {
              selector: w1030 -> [w1046 _]
              tunnel: [w1046 0 ("index of element")] -> w1029
              frame Default {
              }
              frame -1 {
              }
            }
            n403 = case shown="False" w1041 {
              tunnel: [Mode."GetShutterSpeedFpsList" ("Mode") Mode."Error" ("Mode")] -> w1044
              frame False {
              }
              frame True {
              }
            }
            n404 = property on="Frame Rate:" class="Ring (strict)"("Value"=w1029) -> ()  [unwired: 2 in, 2 out]
          }
          frame "SetRecordRate" {
            n405 = property on="Frame Rate:" class="Ring (strict)"() -> ("Strings []"=w1058:string[], "Value"=w1057:u16)  [unwired: 2 in, 2 out]
            n406 = Index Array(array=w1058, index=w1057) -> (element=w1060:string)
            n407 = Match Pattern(string=w1060, regular expression=" fps") -> (before substring=w1056:string)  [unwired: 4 out]
            n408 = Unbundle By Name(w1065) -> ("error"=w1064:errorcluster)
            n409 = Decimal String To Number(string=w1056, default (0L)=u32 0 ("デフォルト (0 I32)")) -> (number=w1054:u32)  [unwired: 2 out]
            n410 = call "PDC_SetRecordRate.vi"("error in (no error)"=w1064, "Rate"=w1054, "ChildNo"=w1053, "DeviceNo"=w1061) -> ("error out"=w1068:errorcluster, "ReturnValue"=w1067:u32, "ErrorCode"=w1062:u32)  [unwired: 5 out]
            n411 = call "Error.vi"("error in (no error)"=w1068, "ErrorCode"=w1062, "ReturnValue"=w1067) -> ("Error_Out"=w1063:T8, "Error?"=w1066:bool)  [unwired: 7 out]
            n412 = case shown="False" w1066 {
              tunnel: [Mode."GetRecordRateList" ("Mode") Mode."Error" ("Mode")] -> w1069
              frame False {
              }
              frame True {
              }
            }
          }
          frame "GetShutterSpeedFpsList" {
            n413 = Unbundle By Name(w1088) -> ("error"=w1087:errorcluster)
            n414 = call "PDC_GetShutterSpeedFpsList.vi"("error in (no error)"=w1087, "ChildNo"=w1076, "DeviceNo"=w1084) -> ("error out"=w1091:errorcluster, "List"=w1081:u32[], "Size"=w1082:u32, "ReturnValue"=w1090:u32, "ErrorCode"=w1085:u32)  [unwired: 4 out]
            n415 = Number To Decimal String(number=w1081, width (-)=u32 0 ("幅（-）")) -> (decimal integer string=w1083:string[])
            n416 = for {
              N: w1082 -> [_]
              tunnel: w1083 -> [w1098]
              tunnel: [w1099] -> w1078 mode=indexing
              tunnel: "1/" -> [w1095]
              tunnel: " sec" -> [w1094]
              i -> [w1097]
              n417 = Index Array(array=w1098, index=w1097) -> (element=w1096:string)
              n418 = Concatenate Strings(w1095, w1096, w1094) -> (w1099:string)
            }
            n419 = call "Error.vi"("error in (no error)"=w1091, "ErrorCode"=w1085, "ReturnValue"=w1090) -> ("Error_Out"=w1086:T8, "Error?"=w1089:bool)  [unwired: 7 out]
            n420 = property on="Shutter:" class="Ring (strict)"("Strings []"=w1078) -> ()  [unwired: 2 in, 2 out]
            n421 = case shown="False" w1089 {
              tunnel: [Mode."GetShutterSpeedFps" ("Mode") Mode."Error" ("Mode")] -> w1092
              frame False {
              }
              frame True {
              }
            }
          }
          frame "GetShutterSpeedFps" {
            n422 = Unbundle By Name(w1118) -> ("error"=w1117:errorcluster)
            n423 = call "PDC_GetShutterSpeedFps.vi"("error in (no error)"=w1117, "ChildNo"=w1105, "DeviceNo"=w1114) -> ("error out"=w1121:errorcluster, "Fps"=w1110:u32, "ReturnValue"=w1120:u32, "ErrorCode"=w1115:u32)  [unwired: 5 out]
            n424 = Number To Decimal String(number=w1110) -> (decimal integer string=w1107:string)  [unwired: 1 out]
            n425 = property on="Shutter:" class="Ring (strict)"() -> ("Strings []"=w1109:string[])  [unwired: 2 in, 2 out]
            n426 = Concatenate Strings("1/", w1107, " sec") -> (w1112:string)
            n427 = Search 1D Array(1D array=w1109, element=w1112) -> (index of element=w1111:i32)  [unwired: 1 out]
            n428 = call "Error.vi"("error in (no error)"=w1121, "ErrorCode"=w1115, "ReturnValue"=w1120) -> ("Error_Out"=w1116:T8, "Error?"=w1119:bool)  [unwired: 7 out]
            n429 = case shown="-1" w1111 {
              selector: w1111 -> [w1124 _]
              tunnel: [w1124 0 ("index of element")] -> w1106
              frame Default {
              }
              frame -1 {
              }
            }
            n430 = property on="Shutter:" class="Ring (strict)"("Value"=w1106) -> ()  [unwired: 2 in, 2 out]
            n431 = case shown="False" w1119 {
              tunnel: [Mode."GetResolutionList" ("Mode") Mode."Error" ("Mode")] -> w1122
              frame False {
              }
              frame True {
              }
            }
          }
          frame "SetShutterSpeedFps" {
            n432 = property on="Shutter:" class="Ring (strict)"() -> ("Strings []"=w1134:string[], "Value"=w1133:u16)  [unwired: 2 in, 2 out]
            n433 = Index Array(array=w1134, index=w1133) -> (element=w1141:string)
            n434 = Match Pattern(string=w1141, regular expression=" sec") -> (before substring=w1138:string)  [unwired: 4 out]
            n435 = Match Pattern(string=w1138, regular expression="1/") -> (after substring=w1136:string)  [unwired: 4 out]
            n436 = Unbundle By Name(w1142) -> ("error"=w1147:errorcluster)
            n437 = Decimal String To Number(string=w1136, default (0L)=u32 0 ("デフォルト (0 I32)")) -> (number=w1135:u32)  [unwired: 2 out]
            n438 = call "PDC_SetShutterSpeedFps.vi"("error in (no error)"=w1147, "Fps"=w1135, "ChildNo"=w1131, "DeviceNo"=w1145) -> ("error out"=w1150:errorcluster, "ReturnValue"=w1149:u32, "ErrorCode"=w1146:u32)  [unwired: 5 out]
            n439 = call "Error.vi"("error in (no error)"=w1150, "ErrorCode"=w1146, "ReturnValue"=w1149) -> ("Error_Out"=w1143:T8, "Error?"=w1148:bool)  [unwired: 7 out]
            n440 = case shown="True" w1148 {
              tunnel: [Mode."GetRecordRateList" ("Mode") Mode."Error" ("Mode")] -> w1144
              frame False {
              }
              frame True {
              }
            }
          }
          frame "GetResolutionList" {
            n441 = Unbundle By Name(w1171) -> ("error"=w1170:errorcluster)
            n442 = call "PDC_GetResolutionList.vi"("error in (no error)"=w1170, "ChildNo"=w1162, "DeviceNo"=w1167) -> ("error out"=w1174:errorcluster, "List"=w1163:u32[], "Size"=w1166:u32, "ReturnValue"=w1173:u32, "ErrorCode"=w1168:u32)  [unwired: 4 out]
            n443 = for {
              N: w1166 -> [_]
              tunnel: " X " -> [w1183]
              tunnel: [w1182] -> w1164 mode=indexing
              tunnel: w1163 -> [w1181]
              tunnel: [w1178] -> w1158 mode=indexing
              tunnel: [w1177] -> w1157 mode=indexing
              i -> [w1180]
              n444 = Index Array(array=w1181, index=w1180) -> (element=w1179:u32)
              n445 = Split Number(x=w1179) -> (hi(x)=w1178:u16, lo(x)=w1177:u16)
              n446 = Number To Decimal String(number=w1178) -> (decimal integer string=w1185:string)  [unwired: 1 out]
              n447 = Number To Decimal String(number=w1177) -> (decimal integer string=w1184:string)  [unwired: 1 out]
              n448 = Concatenate Strings(w1185, w1183, w1184) -> (w1182:string)
            }
            n449 = call "Error.vi"("error in (no error)"=w1174, "ErrorCode"=w1168, "ReturnValue"=w1173) -> ("Error_Out"=w1169:T8, "Error?"=w1172:bool)  [unwired: 7 out]
            n450 = Array Max & Min(array=w1158) -> (max value=w1155:u16)  [unwired: 3 out]
            n451 = Array Max & Min(array=w1157) -> (max value=w1154:u16)  [unwired: 3 out]
            n452 = property on="Resolution:" class="Ring (strict)"("Strings []"=w1164) -> ()  [unwired: 2 in, 2 out]
            n453 = case shown="False" w1172 {
              tunnel: [Mode."GetResolution" ("Mode") Mode."Error" ("Mode")] -> w1175
              frame False {
              }
              frame True {
              }
            }
            n454 = local read "MaxSize"() -> (w1156:cluster{"pWidth":u32, "pHeight":u32})
            n455 = Bundle By Name(cluster=w1156, "pWidth"=w1155, "pHeight"=w1154) -> (→"MaxSize":cluster{"pWidth":u32, "pHeight":u32})
          }
          frame "GetResolution" {
            n456 = Unbundle By Name(w1207) -> ("error"=w1206:errorcluster)
            n457 = call "PDC_GetResolution.vi"("error in (no error)"=w1206, "ChildNo"=w1191, "DeviceNo"=w1203) -> ("error out"=w1210:errorcluster, "Height"=w1192:u32, "Width"=w1193:u32, "ReturnValue"=w1209:u32, "ErrorCode"=w1204:u32)  [unwired: 4 out]
            n458 = Number To Decimal String(number=w1193) -> (decimal integer string=w1200:string)  [unwired: 1 out]
            n459 = Number To Decimal String(number=w1192) -> (decimal integer string=w1201:string)  [unwired: 1 out]
            n460 = call "Error.vi"("error in (no error)"=w1210, "ErrorCode"=w1204, "ReturnValue"=w1209) -> ("Error_Out"=w1205:T8, "Error?"=w1208:bool)  [unwired: 7 out]
            n461 = property on="Resolution:" class="Ring (strict)"() -> ("Strings []"=w1198:string[])  [unwired: 2 in, 2 out]
            n462 = local read "Resolution"() -> (w1195:cluster{"pWidth":u32, "pHeight":u32})
            n463 = Concatenate Strings(w1200, " X ", w1201) -> (w1197:string)
            n464 = Bundle By Name(cluster=w1195, "pWidth"=w1193, "pHeight"=w1192) -> (→"Resolution":cluster{"pWidth":u32, "pHeight":u32})
            n465 = Search 1D Array(1D array=w1198, element=w1197) -> (index of element=w1202:i32)  [unwired: 1 in]
            n466 = case shown="-1" w1202 {
              selector: w1202 -> [w1213 _]
              tunnel: [w1213 0 ("index of element")] -> w1196
              frame Default {
              }
              frame -1 {
              }
            }
            n467 = property on="Resolution:" class="Ring (strict)"("Value"=w1196) -> ()  [unwired: 2 in, 2 out]
            n468 = case shown="False" w1208 {
              tunnel: [w1216 Mode."Error" ("Mode")] -> w1211
              tunnel: w1190 -> [w1215 _]
              frame False {
                n469 = case shown="True" w1215 {
                  tunnel: [Mode."Default" ("Mode") Mode."GetTriggerModeList" ("Mode")] -> w1216
                  frame False {
                  }
                  frame True {
                  }
                }
              }
              frame True {
              }
            }
          }
          frame "SetResolution" {
            n470 = property on="Resolution:" class="Ring (strict)"() -> ("Strings []"=w1230:string[], "Value"=w1229:u16)  [unwired: 2 in, 2 out]
            n471 = Index Array(array=w1230, index=w1229) -> (element=w1236:string)
            n472 = Match Pattern(string=w1236, regular expression=" X ") -> (before substring=w1233:string, after substring=w1231:string)  [unwired: 3 out]
            n473 = Unbundle By Name(w1240) -> ("error"=w1242:errorcluster)
            n474 = Decimal String To Number(string=w1233, default (0L)=u32 0 ("デフォルト (0 I32)")) -> (number=w1226:u32)  [unwired: 2 out]
            n475 = Decimal String To Number(string=w1231, default (0L)=u32 0 ("デフォルト (0 I32)")) -> (number=w1225:u32)  [unwired: 2 out]
            n476 = call "PDC_SetResolution.vi"("DeviceNo"=w1238, "ChildNo"=w1223, "Width"=w1226, "Height"=w1225, "error in (no error)"=w1242) -> ("ReturnValue"=w1244:u32, "ErrorCode"=w1241:u32, "error out"=w1245:errorcluster)  [unwired: 8 out]
            n477 = local read "Resolution"() -> (w1227:cluster{"pWidth":u32, "pHeight":u32})
            n478 = Bundle By Name(cluster=w1227, "pWidth"=w1226, "pHeight"=w1225) -> (w1224:cluster{"pWidth":u32, "pHeight":u32})
            n479 = call "Error.vi"("error in (no error)"=w1245, "ErrorCode"=w1241, "ReturnValue"=w1244) -> ("Error_Out"=w1239:T8, "Error?"=w1243:bool)  [unwired: 7 out]
            n480 = local write "Resolution"(w1224) -> ()
            n481 = case shown="False" w1243 {
              tunnel: [Mode."GetRecordRateList" ("Mode") Mode."Error" ("Mode")] -> w1237
              frame False {
              }
              frame True {
              }
            }
          }
          frame "GetTriggerModeList" {
            n482 = Unbundle By Name(w1260) -> ("error"=w1259:errorcluster)
            n483 = call "PDC_GetTriggerModeList.vi"("error in (no error)"=w1259, "DeviceNo"=w1256) -> ("error out"=w1263:errorcluster, "List"=w1255:u32[], "Size"=w1254:u32, "ReturnValue"=w1262:u32, "ErrorCode"=w1257:u32)  [unwired: 1 in, 4 out]
            n484 = Array Subset(array=w1255, length=w1254) -> (w1252:u32[])  [unwired: 1 in]
            n485 = for {
              tunnel: w1252 -> [w1267] mode=indexing
              tunnel: [w1266] -> w1251 mode=indexing
              n486 = call "GetTrigList.vi"("List"=w1267) -> ("Trigger mode List"=w1266:string)  [unwired: 10 out]
            }
            n487 = call "Error.vi"("error in (no error)"=w1263, "ErrorCode"=w1257, "ReturnValue"=w1262) -> ("Error_Out"=w1258:T8, "Error?"=w1261:bool)  [unwired: 7 out]
            n488 = property on="Trigger Mode:" class="Ring (strict)"("Strings []"=w1251) -> ()  [unwired: 2 in, 2 out]
            n489 = case shown="False" w1261 {
              tunnel: [Mode."GetTriggerMode" ("Mode") Mode."Error" ("Mode")] -> w1264
              frame False {
              }
              frame True {
              }
            }
          }
          frame "GetTriggerMode" {
            n490 = Unbundle By Name(w1283) -> ("error"=w1282:errorcluster)
            n491 = call "PDC_GetTriggerMode.vi"("DeviceNo"=w1279, "error in (no error)"=w1282) -> ("Mode"=w1275:u32, "ReturnValue"=w1285:u32, "ErrorCode"=w1280:u32, "error out"=w1272:errorcluster)  [unwired: 10 out]
            n492 = property on="Trigger Mode:" class="Ring (strict)"() -> ("Strings []"=w1278:string[])  [unwired: 2 in, 2 out]
            n493 = call "GetTrigList.vi"("List"=w1275) -> ("Trigger mode List"=w1274:string)  [unwired: 10 out]
            n494 = Search 1D Array(1D array=w1278, element=w1274) -> (index of element=w1277:i32)  [unwired: 1 out]
            n495 = call "Error.vi"("error in (no error)"=w1272, "ErrorCode"=w1280, "ReturnValue"=w1285) -> ("Error_Out"=w1281:T8, "Error?"=w1284:bool)  [unwired: 7 out]
            n496 = property on="Trigger Mode:" class="Ring (strict)"("Value"=w1277) -> ()  [unwired: 2 in, 2 out]
            n497 = case shown="False" w1284 {
              tunnel: [Mode."GetPartitionList" ("Mode") Mode."Error" ("Mode")] -> w1286
              frame False {
              }
              frame True {
              }
            }
          }
          frame "SetTriggerMode" {
            n498 = property on="Trigger Mode:" class="Ring (strict)"() -> ("Strings []"=w1296:string[], "Value"=w1295:u16)  [unwired: 2 in, 2 out]
            n499 = Index Array(array=w1296, index=w1295) -> (element=w1294:string)
            n500 = case shown="Default" w1294 {
              tunnel: [u32 0 ("nMode") u32 16777216 ("nMode") u32 33554432 ("nMode") u32 67108864 ("nMode") u32 50331648 ("nMode") u32 83886080 ("nMode") u32 100663296 ("nMode") u32 117440512 ("nMode") u32 134217729 ("nMode") u32 134217730 ("nMode") u32 134217731 ("nMode")] -> w1293
              frame Default {
                # "START"
              }
              frame "CENTER" {
                # "CENTER"
              }
              frame "END" {
                # "END"
              }
              frame "RANDOM" {
                # "RANDOM"
              }
              frame "MANUAL" {
                # "MANUAL"
              }
              frame "RANDOM_RESET" {
                # "RANDOM_RESET"
              }
              frame "RANDOM_CENTER" {
                # "RANDOM_CENTER"
              }
              frame "RANDOM_MANUAL" {
                # "RANDOM_MANUAL"
              }
              frame "TWOSTAGE_1/2" {
                # "RANDOM_MANUAL"
              }
              frame "TWOSTAGE_1/4" {
                # "TWOSTAGE_1/4"
              }
              frame "TWOSTAGE_1/8" {
                # "TWOSTAGE_1/8"
              }
            }
            n501 = Unbundle By Name(w1301) -> ("error"=w1303:errorcluster)
            n502 = call "PDC_SetTriggerMode.vi"("DeviceNo"=w1298, "Mode"=w1293, "error in (no error)"=w1303) -> ("ReturnValue"=w1305:u32, "ErrorCode"=w1302:u32, "error out"=w1306:errorcluster)  [unwired: 3 in, 7 out]
            n503 = call "Error.vi"("error in (no error)"=w1306, "ErrorCode"=w1302, "ReturnValue"=w1305) -> ("Error_Out"=w1300:T8, "Error?"=w1304:bool)  [unwired: 7 out]
            n504 = case shown="False" w1304 {
              tunnel: [Mode."Default" ("Mode") Mode."Error" ("Mode")] -> w1299
              frame False {
              }
              frame True {
              }
            }
          }
          frame "GetPartitionList" {
            # "1=NotSupport\n   divided partition"
            n505 = Unbundle By Name(w1335) -> ("error"=w1334:errorcluster)
            n506 = call "PDC_GetPartitionList.vi"("DeviceNo"=w1332, "ChildNo"=w1331, "error in (no error)"=w1334) -> ("ReturnValue"=w1338:u32, "Count"=w1328:u32, "ErrorCode"=w1336:u32, "error out"=w1333:errorcluster)  [unwired: 9 out]
            n507 = To Long Integer(number=w1328) -> (32bit integer=w1322:i32)
            n508 = for {
              N: w1322 -> [_]
              tunnel: "Partition " ("文字列（\"\"）") -> [w1342]
              tunnel: [w1339] -> w1321 mode=indexing
              i -> [w1344]
              n509 = Increment(x=w1344) -> (x+1=w1340:i32)
              n510 = Format Value(string ("")=w1342, format string="%d" ("形式文字列"), value (0)=w1340) -> (output string=w1341:string)
              n511 = Bundle("output string"=w1341, w1340) -> (w1339:cluster{"output string":string, i32})  [unwired: 1 out]
            }
            n512 = call "Error.vi"("error in (no error)"=w1333, "ErrorCode"=w1336, "ReturnValue"=w1338) -> ("Error_Out"=w1330:T8, "Error?"=w1337:bool)  [unwired: 7 out]
            n513 = property on="Partition:" class="Ring (strict)"("StringsAndValues[]"=w1321) -> ()  [unwired: 2 in, 2 out]
            n514 = case shown="False" w1337 {
              tunnel: [Mode."GetCurrentPartition" ("Mode") Mode."Error" ("Mode")] -> w1329
              frame False {
              }
              frame True {
              }
            }
          }
          frame "SetPartitionList" {
            n515 = Unbundle By Name(w1357) -> ("error"=w1356:errorcluster)
            n516 = call "PDC_SetPartitionList.vi"("error in (no error)"=w1356, "ChildNo"=w1353, "DeviceNo"=w1354) -> ("error out"=w1355:errorcluster, "ReturnValue"=w1360:u32, "ErrorCode"=w1358:u32)  [unwired: 2 in, 4 out]
            n517 = call "Error.vi"("error in (no error)"=w1355, "ErrorCode"=w1358, "ReturnValue"=w1360) -> ("Error_Out"=w1352:T8, "Error?"=w1359:bool)  [unwired: 7 out]
            n518 = case shown="False" w1359 {
              tunnel: [Mode."GetCurrentPartition" ("Mode") Mode."Error" ("Mode")] -> w1351
              frame False {
              }
              frame True {
              }
            }
          }
          frame "GetCurrentPartition" {
            # "1=NotSupport\n   divided partition"
            n519 = Unbundle By Name(w1379) -> ("error"=w1378:errorcluster)
            n520 = call "PDC_GetCurrentPartition.vi"("error in (no error)"=w1378, "ChildNo"=w1375, "DeviceNo"=w1376) -> ("error out"=w1377:errorcluster, "No"=w1365:u32, "ReturnValue"=w1382:u32, "ErrorCode"=w1380:u32)  [unwired: 5 out]
            n521 = property on="Partition:" class="Ring (strict)"() -> ("Strings []"=w1368:string[])  [unwired: 2 in, 2 out]
            n522 = Array Size(array=w1368) -> (size(s)=w1367:i32)
            n523 = call "Error.vi"("error in (no error)"=w1377, "ErrorCode"=w1380, "ReturnValue"=w1382) -> ("Error_Out"=w1374:T8, "Error?"=w1381:bool)  [unwired: 7 out]
            n524 = Greater Or Equal?(x=w1367, y=w1365) -> (x >= y?=w1366:bool)
            n525 = Select(t=w1365, s=w1366, f=u32 1) -> (s? t:f=w1363:u32)
            n526 = property on="Partition:" class="Ring (strict)"("Value"=w1363) -> ()  [unwired: 2 in, 2 out]
            n527 = case shown="False" w1381 {
              tunnel: [Mode."GetShadingModeList" ("Mode") Mode."Error" ("Mode")] -> w1373
              frame False {
              }
              frame True {
              }
            }
          }
          frame "SetCurrentPartition" {
            n528 = property on="Partition:" class="Ring (strict)"() -> ("Value"=w1385:u16)  [unwired: 2 in, 2 out]
            n529 = Unbundle By Name(w1391) -> ("error"=w1396:errorcluster)
            n530 = call "PDC_SetCurrentPartition.vi"("error in (no error)"=w1396, "No"=w1385, "ChildNo"=w1392, "DeviceNo"=w1393) -> ("error out"=w1399:errorcluster, "ReturnValue"=w1398:u32, "ErrorCode"=w1395:u32)  [unwired: 5 out]
            n531 = call "Error.vi"("error in (no error)"=w1399, "ErrorCode"=w1395, "ReturnValue"=w1398) -> ("Error_Out"=w1390:T8, "Error?"=w1397:bool)  [unwired: 7 out]
            n532 = case shown="False" w1397 {
              tunnel: [Mode."Default" ("Mode") Mode."Error" ("Mode")] -> w1394
              frame False {
              }
              frame True {
              }
            }
          }
          frame "GetShadingModeList" {
            w1409 = u32 21  # PDC_ERROR_NOT_SUPPORTED
            n533 = Unbundle By Name(w1418) -> ("error"=w1419:errorcluster)
            n534 = call "PDC_GetShadingModeList.vi"("error in (no error)"=w1419, "ChildNo"=w1415, "DeviceNo"=w1416) -> ("error out"=w1421:errorcluster, "List"=w1413:u32[], "Size"=w1412:u32, "ReturnValue"=w1420:u32, "ErrorCode"=w1410:u32)  [unwired: 4 out]
            n535 = Equal?(x=w1410, y=w1409) -> (x = y?=w1408:bool)
            n536 = case shown="False" w1408 {
              tunnel: w1421 -> [w1440 _]
              tunnel: w1420 -> [w1439 _]
              tunnel: [w1438 FALSE ("Error?")] -> w1402
              tunnel: [w1437 T7 {"return type"=1, "pErrorCode"=1, "error "={"status"=FALSE, "code"=0, "source"=""}} ("Error_Out")] -> w1417
              tunnel: w1413 -> [w1436 _]
              tunnel: w1412 -> [w1435 _]
              tunnel: [w1429 u8 2 ("無効")] -> w1411
              tunnel: w1410 -> [w1428 _]
              frame False {
                w1433 = u32 2  # SHADING_ON
                n537 = call "Error.vi"("error in (no error)"=w1440, "ErrorCode"=w1428, "ReturnValue"=w1439) -> ("Error_Out"=w1437:T8, "Error?"=w1438:bool)  [unwired: 7 out]
                n538 = Array Subset(array=w1436, length=w1435) -> (w1434:u32[])  [unwired: 1 in]
                n539 = Search 1D Array(1D array=w1434, element=w1433) -> (index of element=w1432:i32)  [unwired: 1 out]
                n540 = Not Equal?(x=w1432, y=-1) -> (x != y?=w1430:bool)
                n541 = case shown="False" w1430 {
                  tunnel: [u8 2 ("無効") u8 1 ("無効")] -> w1429
                  frame False {
                  }
                  frame True {
                  }
                }
              }
              frame True {
                # "NOT_SUPPORTED ->NO_ERROR"
              }
            }
            n542 = global read "global.vi" "OptionOK"() -> (w1404:bool)
            n543 = case shown="False" w1402 {
              tunnel: [w1425 Mode."Error" ("Mode")] -> w1403
              tunnel: w1404 -> [w1426 _]
              frame False {
                n544 = Select(t=Mode."GetRecordRateList" ("Mode"), s=w1426, f=Mode."Default" ("Mode")) -> (s? t:f=w1425:T2)
                n545 = global write "global.vi" "OptionOK"(FALSE ("OptionOK")) -> ()
              }
              frame True {
              }
            }
            n546 = property on="Shading:" class="Ring (strict)"("Disabled"=w1411) -> ()  [unwired: 2 in, 2 out]
          }
          frame "DataSave" {
            n547 = local read "DataSaveInfo"() -> (w1462:T5)
            n548 = Unbundle By Name(w1467) -> ("error"=w1470:errorcluster)
            n549 = Unbundle By Name(w1462) -> ("StartFrame"=w1459:i32, "EndFrame"=w1458:i32, "DS-Save Path"=w1460:path, "DS-File name:"=w1461:string, "DS-Format"=w1451:u16)
            n550 = case shown="2" w1451 {
              tunnel: [".BMP" ".JPG" ".AVI"] -> w1466
              frame 0, Default {
                # "BMP"
              }
              frame 1 {
                # "JPEG"
              }
              frame 2 {
                # "AVI(Movie)"
              }
            }
            n551 = Bundle("StartFrame"=w1459, "EndFrame"=w1458) -> (w1457:cluster{"StartFrame":i32, "EndFrame":i32})  [unwired: 1 out]
            n552 = Concatenate Strings(w1461, w1466) -> (w1465:string)
            n553 = Build Path(base path=w1460, name or relative path=w1465) -> (appended path=w1450:path)
            n554 = Path To String(path=w1450) -> (string=w1464:string)
            n555 = case shown="2" w1451 {
              tunnel: w1470 -> [w1481 w1489 w1504]
              tunnel: w1468 -> [w1474 w1492 w1496]
              tunnel: w1464 -> [w1472 _ w1501]
              tunnel: w1463 -> [w1475 w1493 w1495]
              tunnel: w1457 -> [_ _ w1499]
              tunnel: [w1479 w1487 w1498] -> w1456
              tunnel: [w1478 w1482 w1497] -> w1455
              tunnel: [w1474 w1492 w1496] -> w1453
              tunnel: [w1475 w1493 w1495] -> w1452
              tunnel: w1450 -> [_ w1486 _]
              tunnel: w1448 -> [w1471 w1485 w1494]
              tunnel: [w1471 w1485 w1494] -> w1447
              frame 0, Default {
                # "BMP"
                n556 = property on="CurrentFrame" class="DigNum (strict)"() -> ("Value"=w1473:i32)  [unwired: 2 in, 2 out]
                n557 = call "PDC_BMPFileSave.vi"("FrameNo"=w1473, "error in (no error)"=w1481, "FileName"=w1472, "ChildNo"=w1474, "DeviceNo"=w1475) -> ("error out"=w1480:errorcluster, "ReturnValue"=w1477:u32, "ErrorCode"=w1476:u32)  [unwired: 4 out]
                n558 = call "Error.vi"("error in (no error)"=w1480, "ErrorCode"=w1476, "ReturnValue"=w1477) -> ("Error_Out"=w1479:T8, "Error?"=w1478:bool)  [unwired: 7 out]
              }
              frame 1 {
                # "ErrorStatus\nCheck"
                # "JPG"
                n559 = local read "Picture"() -> (w1484:picture)
                n560 = call <vilib>:"Picture to Pixmap.vi"("picture"=w1484) -> ("image data"=w1491:T10)  [unwired: 3 in, 7 out]
                n561 = call <vilib>:"Write JPEG File.vi"("quality (80)"=75, "error in (no error)"=w1489, "image data"=w1491, "path to JPEG file"=w1486) -> ("error out"=w1483:errorcluster)  [unwired: 7 out]
                n562 = Unbundle By Name(w1483) -> ("status"=w1482:bool)
                n563 = Bundle By Name(cluster=T7 {"return type"=1, "pErrorCode"=1, "error "={"status"=FALSE, "code"=0, "source"="Write JPEG File.vi"}} ("Error_Out"), "error"=w1483) -> (w1487:T7)
              }
              frame 2 {
                w1503 = 30  # nRate
                # "AVI"
                # "CODEC Dialog"
                n564 = control-ref of="Frame"() -> (w1500:refnum<vi>)
                n565 = call "DataSave.vi"("DeviceNo"=w1495, "FileName"=w1501, "Slide Refnum"=w1500, "ChildNo"=w1496, "Rate"=w1503, "error in (no error)"=w1504, "ShowCompreddDlg"=u32 1 ("nShowCompreddDlg"), "File_Frame"=w1499) -> ("Error?"=w1497:bool, "Error_Out"=w1498:T8)  [unwired: 6 out]
              }
            }
            n566 = case shown="True" w1455 {
              tunnel: [Mode."Default" ("Mode") Mode."Error" ("Mode")] -> w1454
              frame False {
              }
              frame True {
              }
            }
          }
        }
      }
    }
    frame #3 {
      n567 = Quit LabVIEW(quit? (T)=FALSE ("終了?(T)")) -> ()
    }
  }
